vi "AlliGator Phasor Plot Actions.vi"(0 "AlliGator Q Elements in":T4[](array[typedef]), 1 "VI in":refnum<vi>, 2 "Script in":bool, 5 "data value reference in":refnum<data-value>, 7 "AlliGator Q Event in":T5=enum."GUI:Idle", 9 "Data":variant, 11 "error in (no error)":errorcluster, 12 "AlliGator Ctrl Refnums":T6) -> (3 "Script out":bool, 4 "AlliGator Q Elements out":T4[](array[typedef]), 6 "Data Value Reference out":refnum<data-value>, 10 "[Notebook Message]":T1[](array[typedef]) {"Message Style"."Text Alignment" items=["Left", "Right", "Center"]}, 15 "error out":errorcluster)   [LabVIEW 2021, in "AlliGator Action Engine.lvlib"]
doc: "Processes AlliGator phasor plot-related actions."
uses:
  AlliGator Action Engine.lvlib
  Variant/Variant to Data/Variant to Data.lvlib
  Variant/Variant to Data/Variant to [String].vi
  AlliGator Q Event.ctl
  AlliGator Q Element.ctl
  Alligator Elements Order in Action Stack.ctl
  AlliGator Add Single Action to Stack.vi
  GUI/GUI.lvlib
  AlliGator Phasor Plot.lvlib
  AlliGator Phasor Ratio.lvlib
  Variant/Variant to Data/Variant to Boolean.vi
  AlliGator Phasor Plot Color Map.lvlib
  Image/Image.lvlib
  AlliGator Source Image.lvlib
  AlliGator Files.lvlib
  Rich Text Box/Rich Text Box.lvlib
  AlliGator Internal Variables.lvlib
  Files/Files.lvlib
  AlliGator GUI.lvlib
  AlliGator Variables List.ctl
  AlliGator Globals, Variables & Constants.lvlib
  Palette/Palette.lvlib
  Image/Image Display Palette Type.ctl
  Palette/Image Palette Information.ctl
  AlliGator ROI Manager Actions.ctl
  AlliGator ROIs.lvlib
  AlliGator Settings.lvlib
  Utilities/Read-Write.ctl
  Utilities/Utilities.lvlib
  Sound/Sound.lvlib
  <vilib>/Utility/miscctls.llb/LVPoint32TypeDef.ctl
  Image/Image Control Refnum.ctl
  Image/Image Display Mouse Click Event Data.ctl
  Time/Time.lvlib
  Phasor/Phasor (g, s).ctl
  Phasor/Phasor.lvlib
  Variant/Variant to Data/Variant to String.vi
  AlliGator Phasor Plot Image ROI Storage [SGL] v3.vi
  Variant/Variant to Data/Variant to Image.vi
  793a9f64-fd61-4161-b52c-76edb5dbf837.vi
  AlliGator Add Action Array to Stack.vi
  Image/Image Control ROI Description.ctl
  AlliGator Settings List.ctl
  AlliGator Image Display Type.ctl
  Phasor/Phasor Reference Series.ctl
  Phasor/Calibration Phasor (m, phi).ctl
  <vilib>/vision/Image Controls.llb/IMAQ Image.ctl
  Image/Named ROI Description.ctl
  AlliGator Baseline Subtraction Method.ctl
  AlliGator Decay Preprocessing.lvlib
  AlliGator Decay Background Subtraction Info.ctl
  Graphs/XY Graph/XY Graph Plot Shift Method.ctl
  Graphs/XY Graph/XY Graph Add-Ons.lvlib
  Graphs/XY Graph/XY Graph Plot Shift Parameters.ctl
  AlliGator Decay Extrapolation Parameters.ctl
  AlliGator Decay Metadata v3.ctl
  AlliGator Phasor Graph.lvlib
  AlliGator Raw Phasor Plot Data v4.ctl
  AlliGator Data Series Type.ctl
  AlliGator Gate Image Set.ctl
  AlliGator FLI Dataset Type.ctl
  Phasor/Phasor Harmonic Data.ctl
  AlliGator Phasor Multi-Harmonic Data.ctl
  AlliGator Displayed Image.ctl
  Fits/IRF(X)PSED/Decay Fit Parameters & Derived Quantities List.ctl
  Fits/Fits.lvlib
  Fits/IRF(X)PSED/Decay Fit Parameters In List.ctl
  AlliGator Decay Fit Parameter Constraints 2.ctl
  AlliGator Decay Fit.lvlib
  Fits/Decay Convolution/Decay Model.ctl
  Fits/Residual Type.ctl
  Fits/IRF(X)PSED/Fit Weights Type.ctl
  Fits/Fit Calculation Method.ctl
  Fits/Non-linear Fitting Algorithm.ctl
  AlliGator Decay Fit Options & Parameters v2.ctl
  AlliGator Decay Fit Parameter Map.lvlib
  AlliGator Gate Arithmetic.ctl
  AlliGator Internal Variables v2.ctl
  AlliGator Registered Events Ctrl Refnums.ctl
  AlliGator Dataset Ctrl Refnums.ctl
  Phasor/Phasor Calibration Type.ctl
  AlliGator Phasor Graph Ctrl Refnums.ctl
  AlliGator Phasor Plot Ctrl Refnums.ctl
  AlliGator State Indicator.ctl
  AlliGator Other Ctrl Refnums.ctl
  AlliGator Image Histogram Control Refnums.ctl
  AlliGator Decay Fit Map Control Refnums.ctl
  AlliGator Ctrl Refnums.ctl
  Rich Text Box/Text Colors.ctl
  Rich Text Box/Text Formatting.ctl
  AlliGator Dataset Channel.ctl
  AlliGator Dual-Channel Datasets.lvlib
  Histograms/Histogram Bin Position.ctl
  Histograms/Histogram Window.lvlib
  Histograms/Histogram Bin Option.ctl
  Histograms/Linear Histogram Options.ctl
  AlliGator Decay Preprocessing Parameters.ctl
  Phasor/Phasor Standard Deviation Options.ctl
  Phasor/Phasor Calibration Map v2.ctl
  Fits/Non-linear Fitting Method v2.ctl
  Fits/IRF(X)PSED/Decay Fit Options v2.ctl
  Fits/IRF(X)PSED/MLE Baseline Offset Type.ctl
  Notebook/Notebook Message Object.ctl
  Notebook/Notebook.lvlib
  AlliGator Parameter Maps Data.ctl
  AlliGator Main Window Tabs.ctl
panel:
  # "see the AlliGator License on the block diagram (Ctrl+E or Window:Show Block Diagram)"
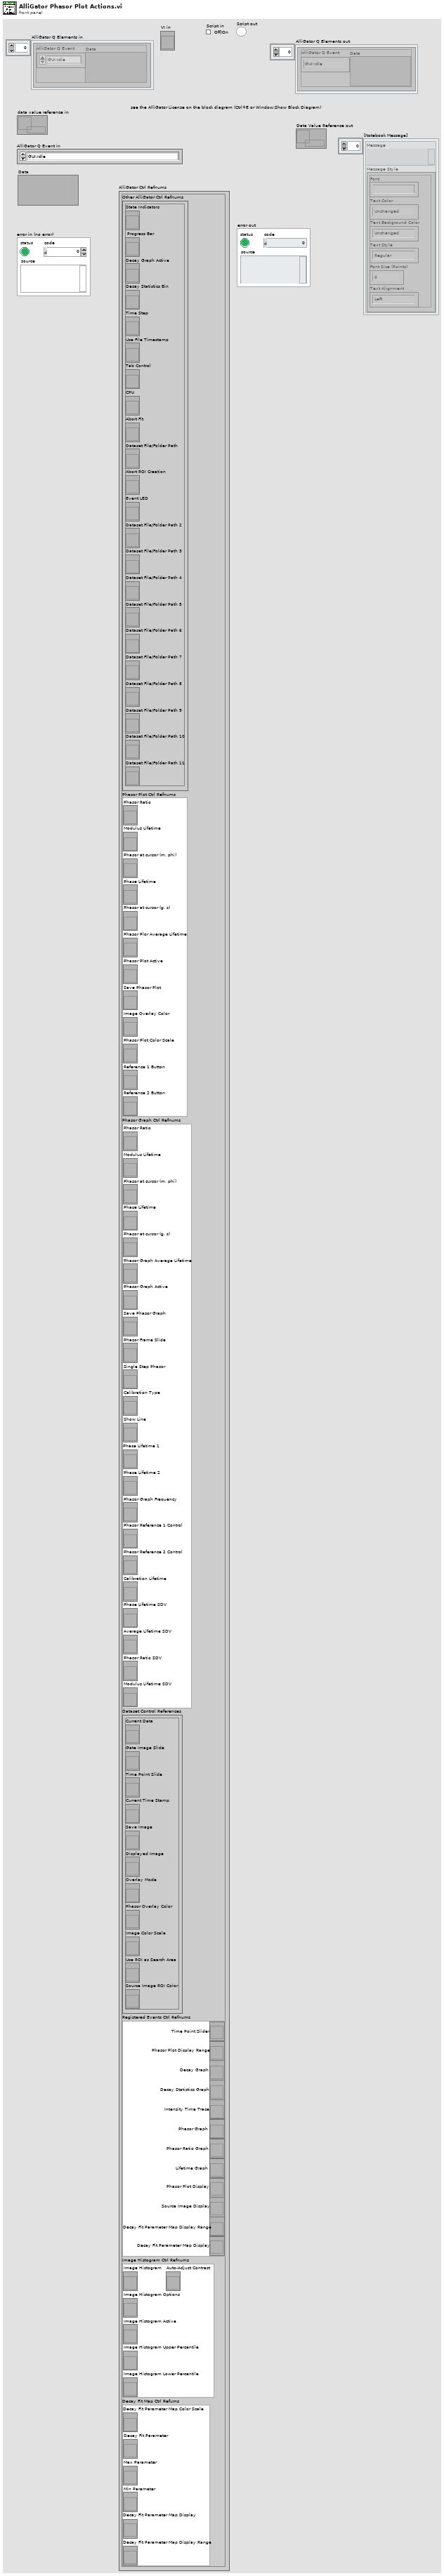
[diagram p1: front panel]
types:
  T1 = typedef "Notebook.lvlib/Notebook Message Object.ctl" = cluster{"Message":string, "Message Style":T2}
  T2 = typedef "Rich Text Box.lvlib/Text Formatting.ctl" = cluster{"Font":string, "Text Color":T3, "Text Background Color":T3, "Text Style":enum16{"Regular", "Bold", "Italic", "Underline", "Strikeout"}, "Font Size (Points)":dbl, "Text Alignment":i32}
  T3 = typedef "Rich Text Box.lvlib/Text Colors.ctl" = enum16{"Unchanged", "Black", "Blue", "Brown", "Gray", "Green", "Orange", "Pink", "Red", "White"}
  T4 = typedef "AlliGator Action Engine.lvlib/AlliGator Q Element.ctl" = cluster{"AlliGator Q Event":T5, "Data":variant}
  T5 = typedef "AlliGator Action Engine.lvlib/AlliGator Q Event.ctl" = enum16{"---- Files ----", "Files:Set Batch Export Files To Save", "Files:Set Dataset Loading & Pre-processing Options", "Files:Check #Frames in Dataset", "Files:Increment Frame Index", "Files:Open Mask Image", "Files:Open White Light Image", "Files:Open Single Dataset", "Files:New Folder of Folders Selected", "Files:Load File (all Types)_Scriptable", "Files:Move Flattened Series to Folders Series", "Files:Select Folder", "Files:Load FLI Dataset", "Files:Load Swiss SPAD 1 Dataset", "Files:Load Swiss SPAD 2 Dataset", "Files:Load .sdt FLI Dataset", "Files:Load .ptu FLI Dataset", "Files:Load .bin FLI Dataset", "Files:Load Single Gate Image Folder", "Files:Load I/m/phi Dataset (deprecated)", "Files:Load Single Image", "Files:Subtract Background File", "Files:Export FLI Dataset", "Files:Load HDF5 FLI Dataset", "Files:Set Destination File Path", "Files:Save Mask Image", "Files:Batch Conversion", "Files:New Folder Selected", "Files:Close FLI Dataset", "Files:Close FLI Dataset Series", "Files:Close White Light Image", "Files:Close Mask Image", "---- FLI Dataset ----", "FLI Dataset:Channel Arithmetic", "FLI Dataset:Export Average Lifetime Map as ASCII", "FLI Dataset:Export User-Defined Quantity Map as ASCII", "FLI Dataset:Python Function FLI Dataset Event", "FLI Dataset:ROI Analysis", "FLI Dataset:Tilted Logistic Square Gated IRF Characteristics Map", "FLI Dataset:Logistic Square Gated IRF Characteristics Map", "FLI Dataset:Square Gated IRF Characteristics Map", "FLI Dataset:Multi-ROI Single-Pixel Phasor Analysis", "FLI Dataset:Multi-ROI Single-Pixel NLSF Analysis", "FLI Dataset:All ROIs IRF Extraction", "FLI Dataset:All ROIs Decay Fit Non-Interactive (Fast + Individual IRF)", "FLI Dataset:All ROIs Phasor Analysis", "FLI Dataset:All ROIs Decay Fit", "FLI Dataset:Fluorescence Decay Statistics", "FLI Dataset:Update Decay Statistics Graph", "FLI Dataset:Get Decay from ROI", "FLI Dataset:All ROIs Average Lifetimes", "---- FLI Dataset Series ----", "FLI Dataset Series:Sum All Datasets in Series", "FLI Dataset Series:Add Dataset to Accumulated Dataset", "FLI Dataset Series:Display Accumulated Dataset", "FLI Dataset Series:Clear Dataset Series Sum", "FLI Dataset Series:Time-Series Analysis (NLSF)", "FLI Dataset Series:Time-Series Analysis (Phasor)", "---- Image ----", "Image:Update Image Profile Plots", "Image:Image Histogram Cursor Move", "Image:Image Histogram", "Image:Image Contrast", "Image:Set Image Histogram Cursor Move Flag", "Image:Clear Image Overlay", "Image:Use ROI as Search Area", "Image:Set ROI Diameter", "Image:Save Image Data as TIFF", "Image:Save Displayed Image with Overlay", "Image:Save Image Overlay Only", "Image:Save Image as Hot Pixel Mask", "Image:Change Source Image Color Palette", "Image:Copy Image to Clipboard", "Image:Source Image ROI Selection", "Image:Delete All ROIs", "Image:Delete All Unselected ROIs", "Image:Delete ROI", "Image:Merge All ROIs", "Image:Store ROI", "Image:Source Image ROI Storage", "Image:Export ROI Description to Notebook", "Image:Save ROI", "Image:Load ROI", "Image:Paste ROI Definition", "Image:Clear ROI", "Image:Identify ROIs in Mask Image", "Image:Create Complementary ROI", "Image:Create Contour ROI", "Image:Create ROI(s) from Pixels with Peak above Min_Scriptable", "Image:Create ROI(s) from Pixels with Intensity above Min_Scriptable", "Image:Compute ROI Statistics", "Image:Delete ROI(s) based on ROI Characteristics", "Image:Create ROI Grid", "Image:ROI to Individual Pixel ROIs", "Image:Python Function Source Image Event", "Image:Show Phasor Calibration Map ROI Centers", "Image:Convert ROI to Mask Image", "Image:Mouse Move", "Image:Mouse Up", "Image:Set Source Image Mouse Move Flag", "Image:Add Scale Bar Overlay", "Image:Delete Existing ROIs Option", "---- Decay ----", "Decay:Clear IRF/Reference Plot", "Decay:Clear Local IRFs", "Decay:Add Decay to Graph", "Decay:Smoothen Plot", "Decay:Smoothen Plot Tail", "Decay:Average Selected Plots", "Decay:Extract IRF", "Decay:Optimal IRF Extraction", "Decay:Threshold IRF", "Decay:Fit to Model IRF", "Decay:Fit IRF to Square Gate", "Decay:Fit IRF to Logistic Square Gate", "Decay:Fit IRF to Tilted Logistic Square Gate", "Decay:Create Bounding Cursors Set", "Decay:Export Bounding Cursors Definition to Notebook", "Decay:Denoise Plot", "Decay:Compute Cumulative Function", "Decay:Use as Reference Decay", "Decay:Show Reference Decay/IRF", "Decay:Extrapolate Decay", "Decay:Create Head & Tail Bounding Cursors", "Decay:Store Cursor-defined Head & Tail Fractions", "Decay:Rebin Plot", "Decay:1-Normalize Decay", "Decay:[0-1]-Normalize Plot", "Decay:Straighten Decay", "Decay:Shift Decay", "Decay:Fold Decay", "Decay:Fit Decay", "Decay:Global Fit of Selected Decays", "Decay:Post Global Fit Script", "Decay:Add Global Fit Parameters to Graph", "Decay:Add Decay Parameter(s) to Plot (Graph)", "Decay:Export Decay to Phasor Graph", "Decay:Plot Decay Shifts", "Decay:Compute Average Lifetime", "Decay:Plot Convolution", "Decay:Graph Tip Strip Update", "---- Decay Statistics ----", "Decay Statistics:Tip Strip Update", "---- Intensity Time Trace ----", "Intensity Time Trace:Use File Timestamp", "Intensity Time Trace:Load Intensity Corrections File", "Intensity Time Trace:Clear Intensity Corrections File", "Intensity Time Trace:Tip Strip Update", "---- Phasor Plot ----", "Phasor Plot:Build Phasor Plot", "Phasor Plot:Change Phasor Plot Color Palette", "Phasor Plot:Adjust Phasor Plot Display Range", "Phasor Plot:Highlight Image ROI in Phasor Plot", "Phasor Plot:Save Phasor Plot Image with Overlay", "Phasor Plot:Export Complex Phasor Map", "Phasor Plot:Export Phasor Ratio Map", "Phasor Plot:Export Average Lifetime Map", "Phasor Plot:Compute Phase Lifetime Histogram", "Phasor Plot:Compute Phasor Ratio Histogram", "Phasor Plot:Compute Phase Lifetime vs Intensity Scatter Plot", "Phasor Plot:Weber 2-Component Decomposition", "Phasor Plot:Update Phasor Color Map Vertices", "Phasor Plot:Clear Phasor Overlay", "Phasor Plot:Use Segment Extremities as References", "Phasor Plot:Use UC/Segment Intersections as References", "Phasor Plot:Use UC/Principal Axis Intersections as References", "Phasor Plot:Use UC/Linear Fit Intersections as References", "Phasor Plot:Update Phasor Plot Reference", "Phasor Plot:Show Local Phasor Info in Phasor Plot", "Phasor Plot:Update Phasor Plot State", "Phasor Plot:Phasor Plot ROI Storage", "Phasor Plot:Phasor Plot ROI Selection", "Phasor Plot:Python Function Phasor Plot Event", "Phasor Plot:Overlay Phasor ROI, Ratio or Map in Source Image", "Phasor Plot:Compute Decay of Selected Phasors", "Phasor Plot:Phasor at Image Pixel", "Phasor Plot:Mouse Move", "Phasor Plot:Mouse Up", "Phasor Plot:Display Range Mouse Move", "Phasor Plot:Set Mouse Move Flag", "---- Phasor Graph ----", "Phasor Graph:Calibrated Phasor Map Series", "Phasor Graph:Whole Image Phasor Scatter Plot (Todo)", "Phasor Graph:Get Phasor Value", "Phasor Graph:Create New Phasor Plot Dialog", "Phasor Graph:Update Last Phasor Value", "Phasor Graph:Update Phasor (m, phi)", "Phasor Graph:Remove Single Phasor from Plot", "Phasor Graph:Add Single Phasor to Plot", "Phasor Graph:Remove Phasor Plot", "Phasor Graph:Remove Selected Phasor Plots", "Phasor Graph:Clear Phasor Data", "Phasor Graph:Clear Phasor Graph", "Phasor Graph:Cursor Move", "Phasor Graph:Draw Cursor Connecting Line", "Phasor Graph:Clear Cursor Connecting Line", "Phasor Graph:Find UC Intersection", "Phasor Graph:Use UC/Cursor-Defined Line Intersections", "Phasor Graph:Use Selected Plots Fitted Line/UC Intersections", "Phasor Graph:Use Selected Plots Principal Axis/UC Intersections", "Phasor Graph:Show Single Phasor", "Phasor Graph:Save Single Phasor Plot", "Phasor Graph:Save All Phasor Plots", "Phasor Graph:Load Phasor Plot(s)", "Phasor Graph:Phasor Multiplication", "Phasor Graph:Compute Average Phasor", "Phasor Graph:Compute Multiple Average Phasors (Selected Plots)", "Phasor Graph:Export Single Phasor Plot Phase Lifetimes", "Phasor Graph:Phase Lifetime Trajectory", "Phasor Graph:Phase Lifetime vs Intensity Scatter Plot (deprecated)", "Phasor Graph:Parameter 2 vs Parameter 1 Scatter Plot", "Phasor Graph:Use Cursor n Location", "Phasor Graph:Set Reference n to Current Phase Lifetime Value", "Phasor Graph:Set Reference n to Lifetime Value", "Phasor Graph:Set Cursor n Location", "Phasor Graph:Save Phasor Graph Image", "Phasor Graph:Update SEPL Plot", "Phasor Graph:Export Single Phasor Plot Data", "Phasor Graph:Export Selected Phasor Plots Data", "Phasor Graph:Python Function Phasor Graph Event", "Phasor Graph:Tip Strip Update", "---- Calibration ----", "Calibration:Set Calibration Type", "Calibration:Load/Save Phasor Calibration", "Calibration:Load/Save Phasor Calibration Series", "Calibration:Load/Save Phasor Calibration Map", "Calibration:Use as Calibration", "Calibration:Compute Optimal Calibration from Phasor References", "Calibration:Clear Phasor Calibration", "Calibration:Single Phasor Calibration Information", "Calibration:Use as Calibration Series", "Calibration:Use as Calibration Map", "Calibration:Clear Calibration Series", "Calibration:Phasor Calibration Series Information", "Calibration:Clear Calibration Map", "Calibration:Phasor Calibration Map Information", "Calibration:Apply Phasor Calibration", "Calibration:Update Single Plot Calibration", "Calibration:Update Multiple Plots Calibration", "Calibration:Clear Single Plot Calibration", "Calibration:Clear All Plots Calibrations", "Calibration:Clear Plot(s) Calibration(s)?", "Calibration:Phasor Calibration Maps (# Gates Series)", "---- Phasor Ratio ----", "Phasor Ratio:Clear Reference n", "Phasor Ratio:Toggle Selected Plot(s)  Lock to Reference 1", "Phasor Ratio:Use as Reference n", "Phasor Ratio:Send Reference n to Notebook", "Phasor Ratio:Toggle Selected Plot(s)  Lock to Reference 2", "Phasor Ratio:Compute Phasor Ratio at Mouse Location", "Phasor Ratio:Compute Phasor Plot's Average Phasor Ratio", "Phasor Ratio:Compute Time-Series Phasor Ratios", "Phasor Ratio:Fit Line to Phasor Ratio Plot", "Phasor Ratio:Save References", "Phasor Ratio:Load References", "Phasor Ratio:Update Phasor Reference 1", "Phasor Ratio:Update Phasor Reference 2", "Phasor Ratio:Move Cursor n to Reference n", "Phasor Ratio:Use as Phasor Reference 1 Lifetime", "Phasor Ratio:Use as Phasor Reference 2 Lifetime", "Phasor Ratio:Export Phasor Ratio Map as ASCII", "Phasor Ratio:Tip Strip Update", "---- Lifetime & Other Parameters Graph ----", "Lifetime:Tip Strip Update", "---- Decay Fit Parameter Map ----", "Decay Fit Parameter Map:Export ROI NLSF Data as ASCII", "Decay Fit Parameter Map:Set Decay Fit  Parameter Map Selection", "Decay Fit Parameter Map:Build Decay Fit Parameter Map", "Decay Fit Parameter Map:Change Decay Fit Parameter Map Color Palette", "Decay Fit Parameter Map:Export Decay Fit Parameter Map Data as ASCII", "Decay Fit Parameter Map:Export All Decay Fit Parameter Maps Data as ASCII", "Decay Fit Parameter Map:Send Map Data to Lifetime Graph", "Decay Fit Parameter Map:Save Decay Fit Parameter Map Image", "Decay Fit Parameter Map:Save-Load IRFs & Fit Data", "Decay Fit Parameter Map:Update Local Decay Plots", "Decay Fit Parameter Map:Python Function Decay Fit Parameters Map Event", "Decay Fit Parameter Map:Overlay Decay Fit Parameter Map in Source Image", "Decay Fit Parameter Map:Plot Map Data vs Intensity", "Decay Fit Parameter Map:Mouse Up", "Decay Fit Parameter Map:Display Range Mouse Move", "---- Generic Graph ----", "Generic Graph:Generic XY Graph Event", "Generic Graph:Python Function XY Graph Event", "Generic Graph:New Plot", "Generic Graph:Save Plot", "Generic Graph:XY Plot Histogram", "Generic Graph:Set XY Graph Plot Name", "Generic Graph:Set Last Cursor Style", "Generic Graph:Tip Strip Update", "---- GUI ----", "GUI:Start Script", "GUI:Type of Displayed Image Changed", "GUI:Gate Image Slide Changed", "GUI:Show Busy Icon", "GUI:Show Busy Icon & Abort Button", "GUI:Hide Busy Icon", "GUI:Hide Busy Icon & Abort Button", "GUI:Abort", "GUI:End Script", "GUI:Start Timing", "GUI:End Timing", "GUI:Set State Indicator", "GUI:Send Parameters JSON Strings to Clipboard", "GUI:Set Gate Step", "GUI:Idle", "GUI:Initialization", "GUI:Quit", "GUI:Increment Dataset Index", "GUI:Set Dataset Index to -1", "GUI:Time Series Slider Moved", "GUI:Time Series Slider Changed", "GUI:Toggle Playback or Loop", "GUI:Playback Script", "GUI:Set Phasor Frequency", "GUI:Open Window", "GUI:Start Test Script", "GUI:End Test Script", "DEBUG"}
  T6 = typedef "AlliGator GUI.lvlib/AlliGator Ctrl Refnums.ctl" = cluster{"Other AlliGator Ctrl Refnums":T7, "Phasor Plot Ctrl Refnums":T8, "Phasor Graph Ctrl Refnums":T9, "Dataset Control References":T10, "Registered Events Ctrl Refnums":T11, "Image Histogram Ctrl Refnums":T12, "Decay Fit Map Ctrl Refums":T13}
  T7 = typedef "AlliGator GUI.lvlib/AlliGator Other Ctrl Refnums.ctl" = cluster{"State Indicators":refnum<vi>, " Progress Bar":refnum<vi>, "Decay Graph Active":refnum<vi>, "Decay Statistics Bin":refnum<vi>, "Time Step":refnum<vi>, "Use File Timestamp":refnum<vi>, "Tab Control":refnum<vi>, "CPU":refnum<vi>, "Abort Fit":refnum<vi>, "Dataset File/Folder Path":refnum<vi>, "Abort ROI Creation":refnum<vi>, "Event LED":refnum<vi>, "Dataset File/Folder Path 2":refnum<vi>, "Dataset File/Folder Path 3":refnum<vi>, "Dataset File/Folder Path 4":refnum<vi>, "Dataset File/Folder Path 5":refnum<vi>, "Dataset File/Folder Path 6":refnum<vi>, "Dataset File/Folder Path 7":refnum<vi>, "Dataset File/Folder Path 8":refnum<vi>, "Dataset File/Folder Path 9":refnum<vi>, "Dataset File/Folder Path 10":refnum<vi>, "Dataset File/Folder Path 11":refnum<vi>}
  T8 = typedef "AlliGator GUI.lvlib/AlliGator Phasor Plot Ctrl Refnums.ctl" = cluster{"Phasor Ratio":refnum<vi>, "Modulus Lifetime":refnum<vi>, "Phasor at cursor (m, phi)":refnum<vi>, "Phase Lifetime":refnum<vi>, "Phasor at cursor (g, s)":refnum<vi>, "Phasor Plor Average Lifetime":refnum<vi>, "Phasor Plot Active":refnum<vi>, "Save Phasor Plot":refnum<vi>, "Image Overlay Color":refnum<vi>, "Phasor Plot Color Scale":refnum<vi>, "Reference 1 Button":refnum<vi>, "Reference 2 Button":refnum<vi>}
  T9 = typedef "AlliGator GUI.lvlib/AlliGator Phasor Graph Ctrl Refnums.ctl" = cluster{"Phasor Ratio":refnum<vi>, "Modulus Lifetime":refnum<vi>, "Phasor at cursor (m, phi)":refnum<vi>, "Phase Lifetime":refnum<vi>, "Phasor at cursor (g, s)":refnum<vi>, "Phasor Graph Average Lifetime":refnum<vi>, "Phasor Graph Active":refnum<vi>, "Save Phasor Graph":refnum<vi>, "Phasor Frame Slide":refnum<vi>, "Single Step Phasor":refnum<vi>, "Calibration Type":refnum<vi>, "Show Line":refnum<vi>, "Phase Lifetime 1":refnum<vi>, "Phase Lifetime 2":refnum<vi>, "Phasor Graph Frequency":refnum<vi>, "Phasor Reference 1 Control":refnum<vi>, "Phasor Reference 2 Control":refnum<vi>, "Calibration Lifetime":refnum<vi>, "Phase Lifetime SDV":refnum<vi>, "Average Lifetime SDV":refnum<vi>, "Phasor Ratio SDV":refnum<vi>, "Modulus Lifetime SDV":refnum<vi>}
  T10 = typedef "AlliGator GUI.lvlib/AlliGator Dataset Ctrl Refnums.ctl" = cluster{"Current Data":refnum<vi>, "Gate Image Slide":refnum<vi>, "Time Point Slide":refnum<vi>, "Current Time Stamp":refnum<vi>, "Save Image":refnum<vi>, "Displayed Image":refnum<vi>, "Overlay Mode":refnum<vi>, "Phasor Overlay Color":refnum<vi>, "Image Color Scale":refnum<vi>, "Use ROI as Search Area":refnum<vi>, "Source Image ROI Color":refnum<vi>}
  T11 = typedef "AlliGator GUI.lvlib/AlliGator Registered Events Ctrl Refnums.ctl" = cluster{"Time Point Slider":refnum<vi>, "Phasor Plot Display Range":refnum<vi>, "Decay Graph":refnum<vi>, "Decay Statistics Graph":refnum<vi>, "Intensity Time Trace":refnum<vi>, "Phasor Graph":refnum<vi>, "Phasor Ratio Graph":refnum<vi>, "Lifetime Graph":refnum<vi>, "Phasor Plot Display":refnum<vi>, "Source Image Display":refnum<vi>, "Decay Fit Parameter Map Display Range":refnum<vi>, "Decay Fit Parameter Map Display":refnum<vi>}
  T12 = typedef "AlliGator GUI.lvlib/AlliGator Image Histogram Control Refnums.ctl" = cluster{"Image Histogram":refnum<vi>, "Image Histogram Options":refnum<vi>, "Image Histogram Active":refnum<vi>, "Image Histogram Upper Percentile":refnum<vi>, "Image Histogram Lower Percentile":refnum<vi>, "Auto-Adjust Contrast":refnum<vi>}
  T13 = typedef "AlliGator Decay Fit Parameter Map.lvlib/AlliGator Decay Fit Map Control Refnums.ctl" = cluster{"Decay Fit Parameter Map Color Scale":refnum<vi>, "Decay Fit Parameter":refnum<vi>, "Max Parameter":refnum<vi>, "Min Parameter":refnum<vi>, "Decay Fit Parameter Map Display":refnum<vi>, "Decay Fit Parameter Map Display Range":refnum<vi>}
  T14 = typedef "AlliGator Action Engine.lvlib/Alligator Elements Order in Action Stack.ctl" = enum16{"Enqueue 2 AFTER 1", "Enqueue 2 BEFORE 1"}
  T15 = typedef "Image.lvlib/AlliGator Image Display Type.ctl" = enum16{"Source Image", "Phasor Plot", "Decay Fit Parameter Map"}
  T16 = typedef "AlliGator Globals, Variables & Constants.lvlib/AlliGator Variables List.ctl" = enum16{"---- GUI ----", "GUI:Initialization Status", "GUI:State Indicators Refnum", "GUI:Original AlliGator Menu Items", "GUI:Current Action Loop State", "GUI:Script in progress", "GUI:Playback", "GUI:Loop Playback", "GUI:Search ROI Used", "GUI:Search ROI", "Decay Graph Max Legend Size", "Intensity Graph Max Legend Size", "Decay Statistics Graph Max Legend Size", "Phasor Graph Max Legend Size", "Phasor Ratio Graph Max Legend Size", "Lifetime Graph Max Legend Size", "---- Files ----", "Files:Export Dataset Frames as Individual Files", "Files:Show Batch Export Help Balloons", "Files:Frames in Dataset", "Files:ptu File Frame Start Indices", "Files:Current Frame in Dataset", "Files:Current Frame Timestamp", "Files:Dataset Loaded", "Files:Dataset Metadata", "Files:Dataset Channel", "Files:Dataset Data Description", "Files:Background Dataset Metadata", "Files:Background Dataset Channel", "Files:Background Dataset Data Description", "Files:Background File Subtraction", "Files:Background File Path", "Files:Background File Pile-up Correction", "Files:Background File Pixel Well Capacity", "Files:Background File Scaling Factor", "Files:Current Dataset Load Settings", "Files:Dataset Path", "Files:ICCD-specific Information", "Files:Macrotime Gate Separation", "------ Python Plugins ------", "Python Plugins:Information", "Python Plugins:Python Session", "Python Plugins:Valid Python Session?", "---- Source Image ----", "Source Image:ROIs", "Source Image:Current ROI", "Source Image:ROI Event Refnum", "X_Source Image Display Range", "X_Source Image Palette Information", "X_Type of Displayed Image", "X_Time Gate Slider", "Source Image:Palette List", "Source Image:Scale", "Source Image:ROI Overlay Color", "Source Image:Overlay to Erase", "Source Image:Is Displayed Image Accumulated", "---- Image Profile Window ----", "Image Profile:Overlay ROI in Source Image", "Image Profile:Window Event Refnum", "Image Profile:IntensityType", "Image Profile:Intensity Average Type", "Image Profile:Intensity-weighted SDV", "Image Profile:Box Profile Type", "Image Profile:Window Open", "Image Profile:Plotted Fit Parameter", "Source Image:White Light Image Modified", "Source Image:Mask Image Modified", "------ Phasor Graph -------", "Phasor Graph:Show Line", "---- Phasor Plot ---", "Phasor Plot:Parameters Changed", "Phasor Plot:FLI Dataset Modified since last Calculation", "Phasor Harmonics Data", "Selected Phasor Harmonics", "Phasor Harmonic Manager Event Refnum", "Phasor Plot:ROIs", "Phasor Plot::Current ROI", "Phasor Plot:ROI Event Refnum", "Phasor Plot:Image Reference Points", "Phasor Plot:Computed", "Phasor Plot:Palette Information", "Phasor Plot:Palette List", "Phasor Ratio Palette Information", "Phasor Ratio Palette List", "Phasor Plot:Image Scale", "Phasor Plot:Image Overlay to Erase", "Phasor Plot:Image Elements to Update", "Current Phasor Plot Calculation Parameters", "Current Phasor Calibration Options", "Phasor Plot:Reset Cumulated Phasor Plot", "Phasor Plot:Reference 1", "Phasor Plot:Lifetime Reference 1", "Phasor Plot:Reference 1 Frequency", "Phasor Plot:Reference 2", "Phasor Plot:Lifetime Reference 2", "Phasor Plot:Reference 2 Frequency", "---- Decay Analysis ----", "Number of Selected Decays to Fit", "LS Fit Results", "LAR Fit Results", "BS Fit Results", "Last Decay Max - Min", "Best Fit Parameters", "Best Fit Parameter Names", "Actual Size X", "Actual Size Y", "Binning X", "Binning Y", "Actual # Gates", "Dataset Number", "Gates to...", "Gates Skipped", "Gates to keep", "Gate Step", "Gate Separation", "Reversed Gates", "Pile-up Correction", "Pixel Well Capacity", "Background Subtracted", "Background Subtraction Method", "Background Definition Range", "Background File (deprecated)", "Number of Dataset Accumulated", "Array of Accumulated Dataset Paths", "Do Averaged Datasets", "Destination File Path", "Process Plot Target", "Use 1/D as Phasor Frequency", "---- Decay Fit Parameter Map -----", "Decay Fit Parameter Map Palette Information", "Decay Fit Parameter Map Palette List", "Local Decay Graph Window Event Refnum", "------- Local Decay Window ---------", "Use normalized IRF for convolution", "----- Miscellaneous ----", "Skippable Dialog Windows Status"}
  T17 = typedef "Palette.lvlib/Image Palette Information.ctl" = cluster{"Palette Name [# Colors,int?,inv?]":string, "Palette Type":T18, "Palette Colors":u32[], "Interpolate?":bool}
  T18 = typedef "Image.lvlib/Image Display Palette Type.ctl" = u32
  T19 = typedef "AlliGator Settings.lvlib/AlliGator Settings List.ctl" = enum16{"GUI:Visible Settings Tab", "GUI:Last Run Version", "Source Image:Use Image Histogram for Contrast", "Source Image:Low Count Pixels Rejection Options", "Source Image:High Count Pixels Rejection Options", "Source Image:Use Image Brightness", "Source Image:Blend Overlay with Image Background", "Source Image:Use Fixed ROI Diameter", "Source Image:ROI Diameter", "Source Image:ROI Center Color", "Source Image:Peak Threshold", "Source Image:Intensity Threshold", "Source Image:Image Binning Options", "Source Image:Image Smoothing Options", "Source Image:Image Histogram Active", "Source Image:Invert Binary Mask", "Source Image:Hot Pixel Removal", "Source Image:Overlay Analyzed ROI Center", "Source Image:Auto-Adjust Contrast", "Source Image:Histogram Lower Percentile", "Source Image:Histogram Upper Percentile", "Source Image:Save Source Image", "Source Image:Scale Bar Options", "Source Image:Image Resolution (Pixel Size)", "Source Image:Flatfield Correction", "Source Image:Show Dead Left Columns Correction", "Source Image:Dead Left Columns Correction", "Source Image:Image Pre-Processing Operations Order", "Data Information:Gate Width", "Data Information:Nanotime Gate Separation", "Data Information:Macrotime Gate Separation", "Data Information:Gate Step", "Data Information:# Gates", "Data Information:Gate Image Exposure", "Data Information:Gate Image Integration", "Data Information:Gates to Skip", "Data Information:Gates to Keep", "Data Information:Define Gates to", "Data Information:Channel Name", "Data Information:Available Channel Names", "Data Information:Channel Arithmetic", "Data Information:Background File Subtraction", "Data Information:Background File", "Data Information:Background Scaling Factor", "Data Information:Background Pile-up Correction", "Data Information:Background Pixel Well Capacity", "Data Information:Laser Period", "Data Information:SYNC Period", "Data Information:Pile-up Correction", "Data Information:Pixel Well Capacity", "Data Information:Dataset Scaling Factor", "Fluorescence Decay_Decay Pre-Processing:Reverse Gates", "Fluorescence Decay_Decay Pre-Processing:Verbose Decay Pre-Processing", "Fluorescence Decay_Decay Pre-Processing:Use Decay Pre-Processing", "Fluorescence Decay_Decay Pre-Processing:Background Subtraction", "Fluorescence Decay_Decay Pre-Processing:Background Definition Range", "Fluorescence Decay_Decay Pre-Processing:Baseline Subtraction Method", "Fluorescence Decay_Decay Pre-Processing:Decay Pre-Processing Operations Order", "Fluorescence Decay_Decay Pre-Processing:Smoothing Parameter", "Fluorescence Decay_Decay Pre-Processing:Shift Decay", "Fluorescence Decay_Decay Pre-Processing:Decay Shift Parameters", "Fluorescence Decay_Decay Pre-Processing:Fold Decay", "Fluorescence Decay_Decay Pre-Processing:# Folds", "Fluorescence Decay_Decay Pre-Processing:1-Normalize Decay", "Fluorescence Decay_Decay Pre-Processing:[0-1]-Normalize Decay", "Fluorescence Decay_Decay Pre-Processing:Smoothen Decay", "Fluorescence Decay_Decay Pre-Processing:Extrapolate Decay", "Fluorescence Decay_Decay Pre-Processing:Use Periodicity", "Fluorescence Decay_Decay Pre-Processing:Use Cursors", "Fluorescence Decay_Decay Pre-Processing:Tail Fraction", "Fluorescence Decay_Decay Pre-Processing:Head Fraction", "Fluorescence Decay_Decay Pre-Processing:Additional Points", "Fluorescence Decay_Decay Pre-Processing:Straighten Decay", "Fluorescence Decay_Decay Pre-Processing:Constant Background", "Fluorescence Decay_Decay Pre-Processing:Pixel-Normalize Decay", "Fluorescence Decay_Advanced Analysis:Extract IRF instead of Decay", "Fluorescence Decay_Advanced Analysis:IRF Extraction Options", "Fluorescence Decay_Advanced Analysis:IRF Optimization Options", "Fluorescence Decay_Advanced Analysis:Square Pulse Options", "Fluorescence Decay_Advanced Analysis:IRF Order", "Fluorescence Decay_Advanced Analysis:IRF Time Constants", "Fluorescence Decay_Advanced Analysis:Wavelet Analysis Options", "Fluorescence Decay_Advanced Analysis:Average Lifetime Options", "Fluorescence Decay_Fit Options:Fit Options", "Fluorescence Decay_Fit Options:Use Legacy Fitting Approach", "Fluorescence Decay_Fit Options:Use Data Information Laser Period", "Fluorescence Decay_Fit Parameters:Displayed Fit Parameters", "Fluorescence Decay_Fit Parameters:Fit Parameter Constraints", "Fluorescence Decay_Fit Parameters:Export Tabulated Results", "Fluorescence Decay_Fit Parameters:MLE Baseline Offset Type", "Fluorescence Decay_Fit Parameters:MLE Baseline Offset", "Fluorescence Decay_Fit Parameters:Guess Parameter Names", "Fluorescence Decay_Fit Parameters:Guess Parameter Values", "Fluorescence Decay_Fit Parameters:Guess Parameters Options", "Fluorescence Decay_Styles:Show Last Decay Only", "Fluorescence Decay_Styles:Decay Graph Color Array", "Fluorescence Decay:Decay Graph Active", "Fluorescence Decay Statistics:Min Peak Value", "Fluorescence Decay Statistics:Reject Low Decay Peak Pixels", "Fluorescence Decay Statistics:Reject High Decay Peak Pixels", "Fluorescence Decay Statistics:Max Peak Value", "Time Traces:Use File Timestamp", "Time Traces:Time Step", "Time Traces:Use Intensity Correction File", "Time Traces:Intensity Correction File", "Phasor Plot:Phasor Plot Smoothing Options", "Phasor Plot:Phasor Plot Size", "Phasor Plot:Phasor Plot Graphics Options", "Phasor Plot:Cumulative Phasor Plot", "Phasor Plot:Use Phasor Brightness", "Phasor Plot:Blend Overlay with Phasor Background", "Phasor Plot:Save Phasor Plot", "Phasor Plot:Show References", "Phasor Plot:Phasor Ratio Decay Range", "Phasor Plot:Exponential Fading", "Phasor Plot:Phasor Ratio Reference Colors", "Phasor Plot:Reference Radius", "Phasor Plot:Show Color Map Vertices", "Phasor Plot:Phasor Plot Active", "Phasor Plot:Phasor Ratio Color Map Type", "Phasor Plot:Phasor Ratio Color Map", "Phasor Plot:Phasor Ratio Display Range", "Phasor Plot:Selected Image ROI(s)", "Phasor Plot:All Image ROIs", "Phasor Plot:Selected Phasor Plot ROI(s)", "Phasor Plot:All Phasor Plot ROIs", "Phasor Plot:Phasor Ratio Color-Coded Quantity", "Phasor Plot:Store Phasor Harmonics", "Phasor Plot:Draw Reference Segment", "Phasor Plot:User-Defined Quantity", "Phasor Graph:Phasor Frequency", "Phasor Graph:Phasor Ratio Type", "Phasor Graph:Pixel-level Phasor Computation", "Phasor Graph:Save Phasor Graph", "Phasor Graph:Phasor Graph Active", "Phasor Graph:Phasor SDV Options", "Phasor Calibration:Use Backup Calibration if needed", "Phasor Graph:Define Shortest Lifetime as", "Phasor Calibration:Backup Calibration Type", "Phasor Calibration:Calibration Type", "Phasor Calibration:Calibration Lifetime", "Phasor Calibration:Calibration Map Algorithm", "Single-Exponential Phasor Locus (SEPL):Gate Parameters", "Single-Exponential Phasor Locus (SEPL):User-defined Gate", "Single-Exponential Phasor Locus (SEPL):User-defined IRF", "Single-Exponential Phasor Locus (SEPL):Phasor Parameters", "Single-Exponential Phasor Locus (SEPL):Decay & IRF Parameters", "Single-Exponential Phasor Locus (SEPL):Display Parameters", "Lifetime Analysis:Decay Analysis Parameters", "Lifetime Analysis:Lifetime Map Active", "Plugins:Python Settings", "Miscellaneous:Verbose Mode", "Miscellaneous:Beep after Script", "Miscellaneous:Saved Image File Format", "Miscellaneous:Exported Gate Image Settings", "Miscellaneous:Include Loading in Timing", "Miscellaneous:Verbose Settings Mode", "Miscellaneous:Histogram Options", "Miscellaneous:Beep on Error", "Miscellaneous:# Logical Processors Used", "Miscellaneous:ROI Description Max Characters", "Miscellaneous:Verbose Error Mode", "Miscellaneous:Transparent Mask Color"}
  T20 = typedef "Image.lvlib/Image Control ROI Description.ctl" = cluster{"Image Control Label":string, "ROI Descriptor":T21}
  T21 = typedef "ROI Descriptor" = cluster{"Global Rectangle":i32[], "Contours":cluster{"ID":enum32{"External", "Internal"}, "Type":u32, "Coordinates":i32[]}[]}
  T22 = typedef "Image.lvlib/Image Display Mouse Click Event Data.ctl" = cluster{"Image Control Refnum":T23, "Mouse Coordinates":T24}
  T23 = typedef "Image.lvlib/Image Control Refnum.ctl" = refnum<vi>
  T24 = typedef "LVPoint32TypeDef.ctl" = cluster{"Horizontal":i32, "Vertical":i32}
  T25 = typedef "AlliGator ROIs.lvlib/AlliGator ROI Manager Actions.ctl" = enum16{"Undefined", "Delete Current ROI", "Delete All Unselected ROIs", "Delete Multiple ROIs", "Delete All ROIs", "Swap ROIs", "Insert ROI", "Update Current ROI Descriptor", "Rename Current ROI", "Store New ROI", "Store Multiple ROIs", "Select Next ROI", "Select Previous ROI", "Find Selected ROI", "Show All ROIs", "Update ROI Manager Window", "Merge All ROIs", "Unmerge ROI", "Set Selected ROI by ID"}
  T26 = typedef "Utilities.lvlib/Read-Write.ctl" = enum16{"Read", "Write"}
  T27 = typedef "Phasor.lvlib/Phasor (g, s).ctl" = cluster{"g":dbl, "s":dbl}
  T28 = typedef "AlliGator GUI.lvlib/AlliGator State Indicator.ctl" = cluster{"Phasor Calibration Defined":bool, "Phasor Calibration Series Defined":bool, "Phasor Calibration Map Defined":bool, "Phasor Ratio Reference 1 Defined":bool, "Phasor Ratio Reference 2 Defined":bool, "Phasor Ratio Lifetime Reference 1 Defined ":bool, "Phasor Ratio Lifetime Reference 2 Defined":bool, "Phasor Calibration Used":bool, "Phasor Calibration Series Used":bool, "Phasor Calibration Map Used":bool, "Dataset Update Needed":bool, "Phasor Plot Update Needed":bool, "Reference/IRF Defined":bool, "Individual IRFs Defined":bool}
  T29 = typedef "Image.lvlib/Image Display User Event Data.ctl" = cluster{"Image Control Refnum":T23, "Coords":T24, "button info":cluster{"button 1":bool, "button 2":bool, "button 3":bool, "button 4":bool}, "keys pressed":enum16{"0", "1", "2", "3", "4", "5", "6", "7", "8", "9", "A", "B", "C", "D", "E", "F", "G", "H", "I", "J", "K", "L", "M", "N", "O", "P", "Q", "R", "S", "T", "U", "V", "W", "X", "Y", "Z", "F1", "F2", "F3", "F4", "F5", "F6", "F7", "F8", "F9", "F10", "F11", "F12", "F13", "F14", "F15", "ADD", "BACK", "BACKSLASH", "CAPITAL", "COMMA", "DECIMAL", "DELETE", "DIVIDE", "DOWN", "END", "EQUALS", "ESCAPE", "GRAVE (`)", "HOME", "INSERT", "LBRACKET", "LCONTROL", "LEFT", "L ALT", "LSHIFT", "LWIN", "MINUS", "MULTIPLY", "NEXT", "NUMLOCK", "NUMPAD_0", "NUMPAD_1", "NUMPAD_2", "NUMPAD_3", "NUMPAD_4", "NUMPAD_5", "NUMPAD_6", "NUMPAD_7", "NUMPAD_8", "NUMPAD_9", "PAUSE", "PERIOD", "PRIOR (PG UP)", "RBRACKET", "RCONTROL", "RETURN", "RIGHT", "R ALT", "RSHIFT", "RWIN", "SCROLL", "SEMICOLON", "SLASH", "SPACE", "SUBTRACT", "TAB", "UP", "ENTER (num pad)", "' (quote)"}[]}
  T30 = typedef "AlliGator Phasor Plot.lvlib/AlliGator Phasor Plot Mouse Up Event Data.ctl" = cluster{"Current ROI Tool":u32, "ROI Descriptor":T31, "Shift":bool, "Alt":bool}
  T31 = typedef "Image.lvlib/Image ROI Descriptor.ctl" = cluster{"Global Rectangle":i32[], "Contours":T32[]}
  T32 = typedef "Image.lvlib/Image Contour Definition.ctl" = cluster{"Contour Type":T33, "ROI Type":T34, "Points":i32[]}
  T33 = typedef "Image.lvlib/Image Contour ID.ctl" = enum32{"External", "Internal"}
  T34 = typedef "Image.lvlib/Image ROI Type.ctl" = enum16{"No Selection", "Point", "Line", "Rectangle", "Oval", "Polygon", "Freehand Region", "Annulus", "Unused2", "Unused3", "Broken Line", "Freehand Line", "Rotated Rectangle"}
  T35 = typedef "Image.lvlib/Image Color Scale Information.ctl" = cluster{"Scale.Maximum":dbl, "Scale.Minimum":dbl, "Scale.High Color":u32, "Scale.Low Color":u32}
  T36 = typedef "IMAQ Image.ctl" = refnum<image>
  T37 = cluster{"Global Rectangle":i32[], "Contours":cluster{"Contour Type":u32, "ROI Type":u32, "Points":i32[]}[]}
  T38 = typedef "Image.lvlib/Image Save File Format.ctl" = enum16{"PNG", "JPEG", "BMP"}
  T39 = typedef "Image.lvlib/Image Point.ctl" = cluster{"X":i32, "Y":i32}
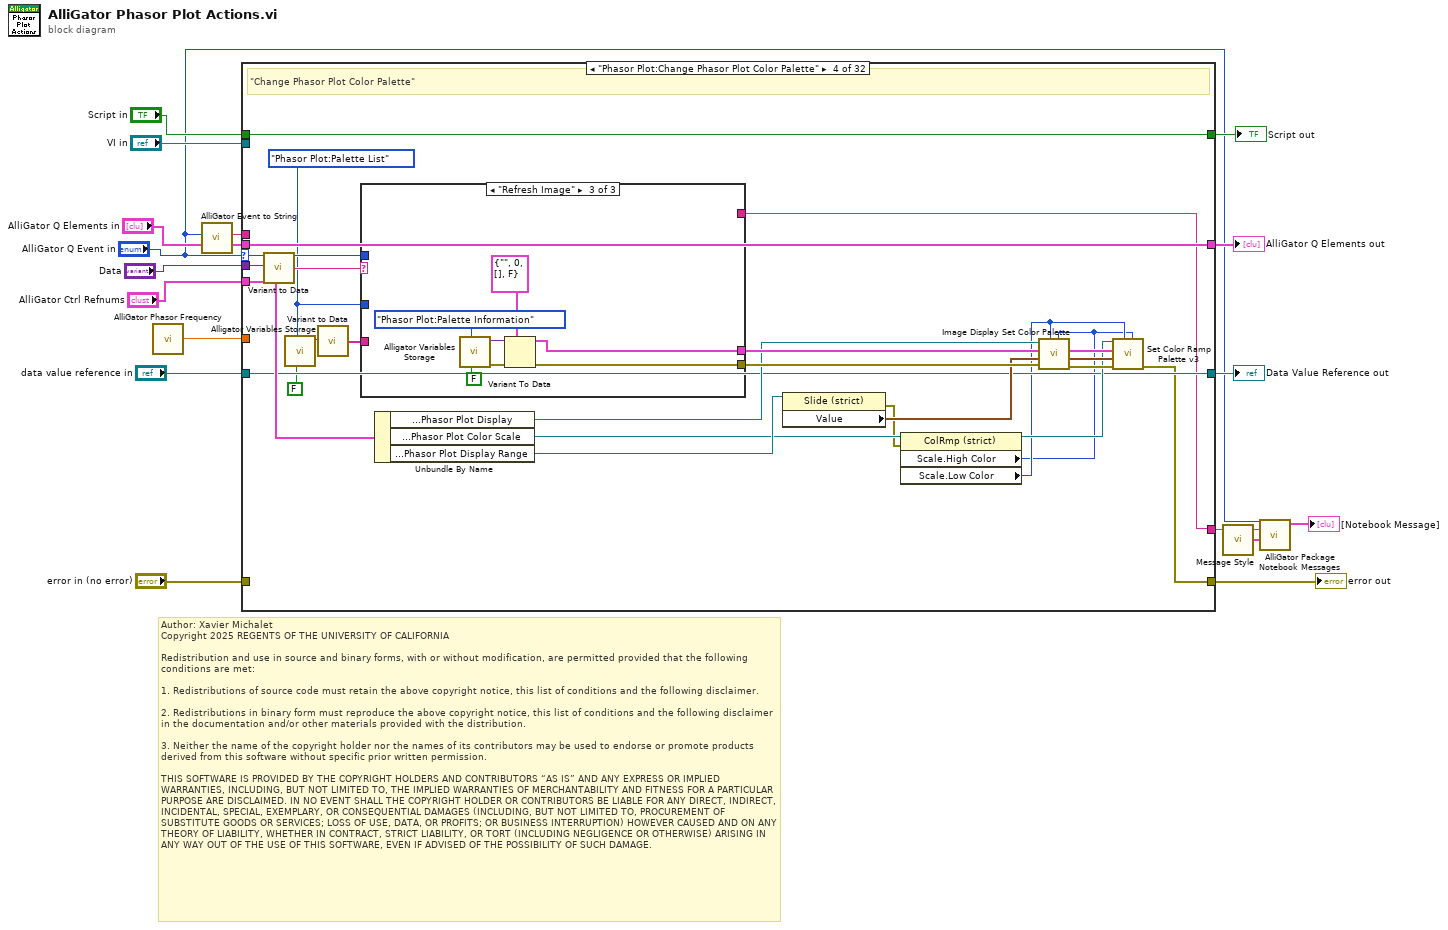
[diagram p0: block diagram]
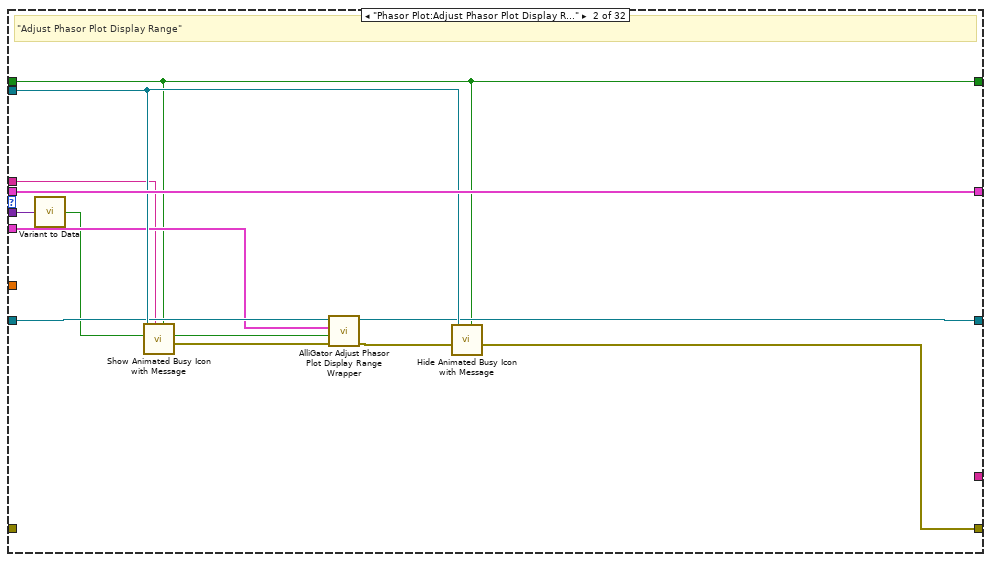
[diagram p3: hidden frame]
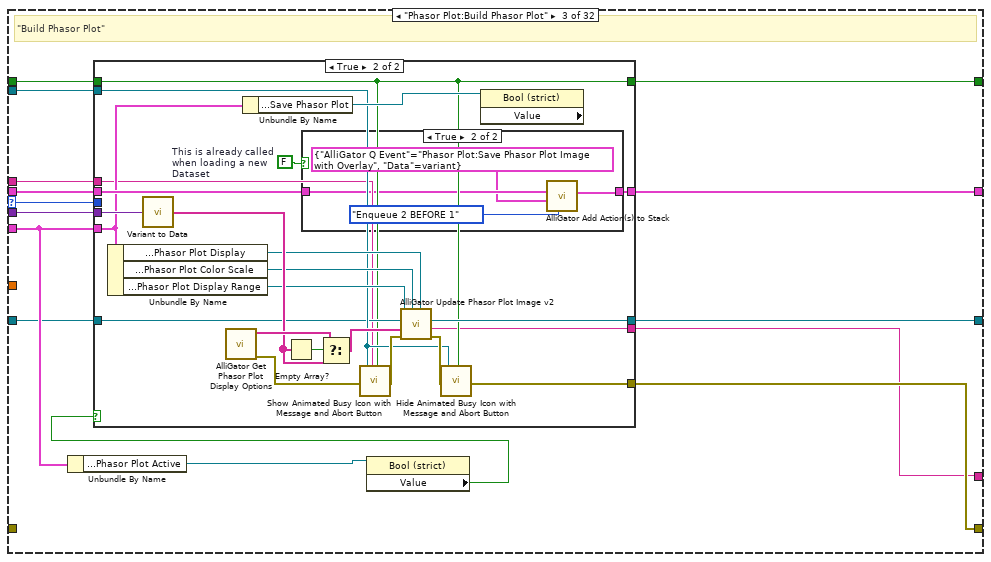
[diagram p4: hidden frame]
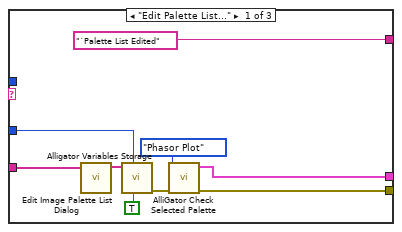
[diagram p7: hidden frame]
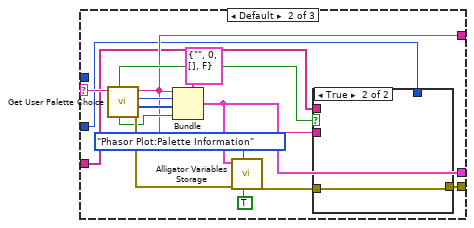
[diagram p8: hidden frame]
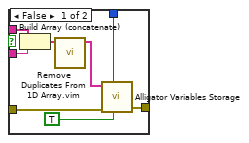
[diagram p9: hidden frame]
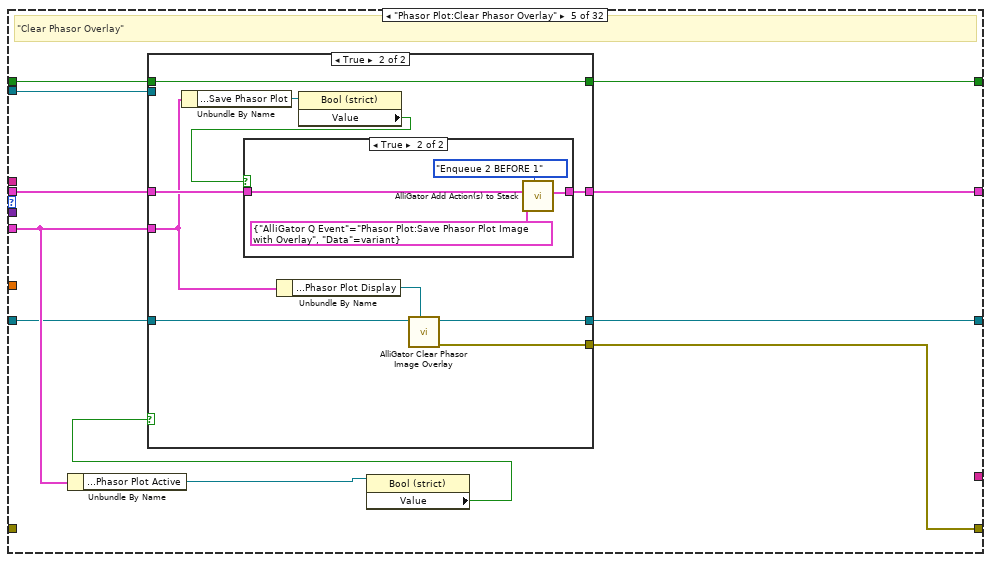
[diagram p10: hidden frame]
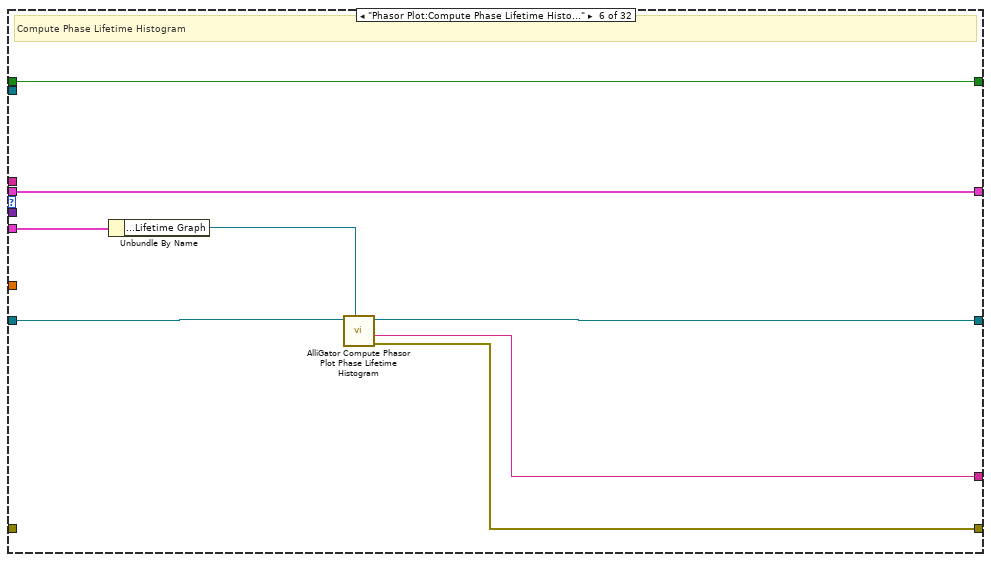
[diagram p13: hidden frame]
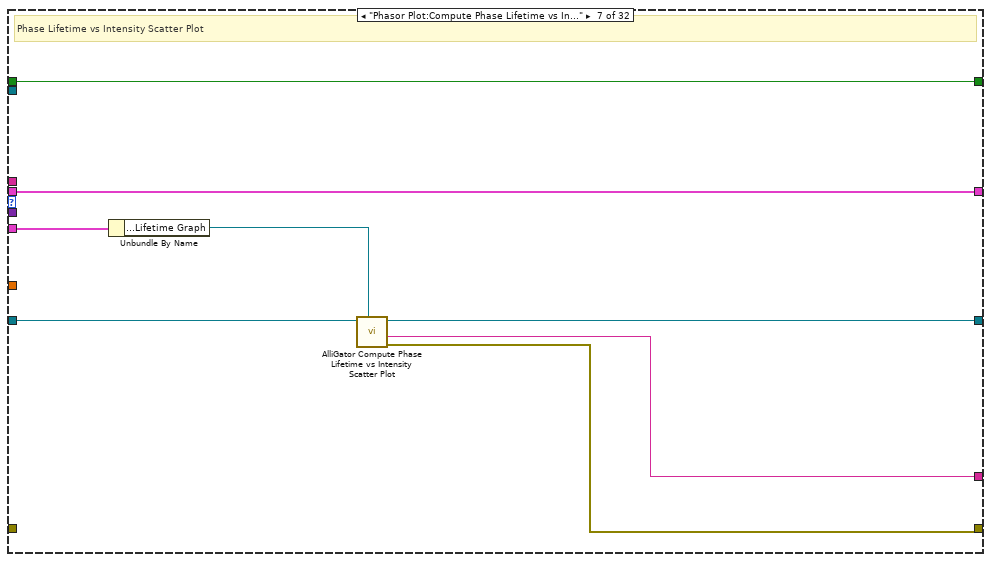
[diagram p14: hidden frame]
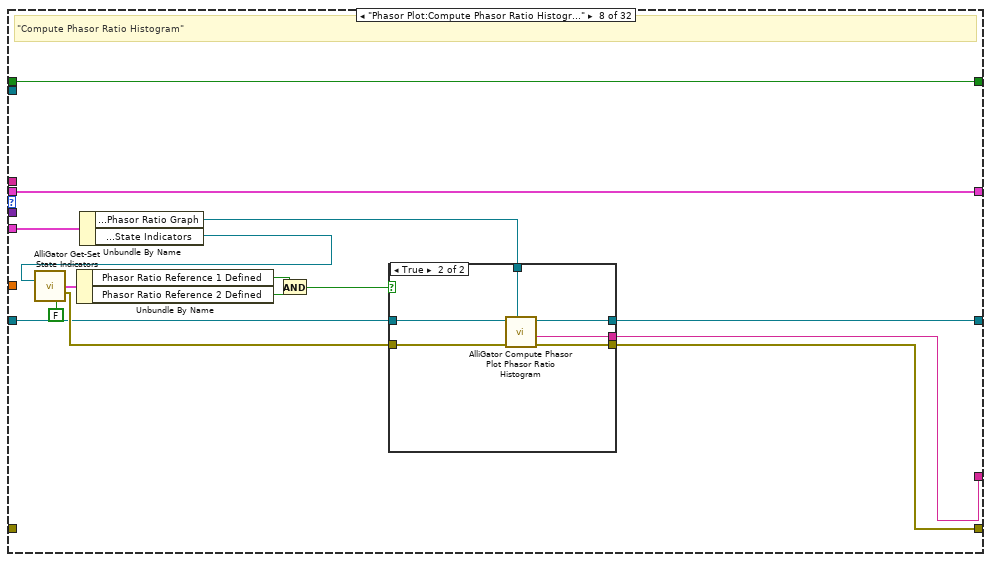
[diagram p15: hidden frame]
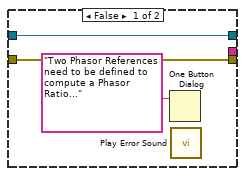
[diagram p16: hidden frame]
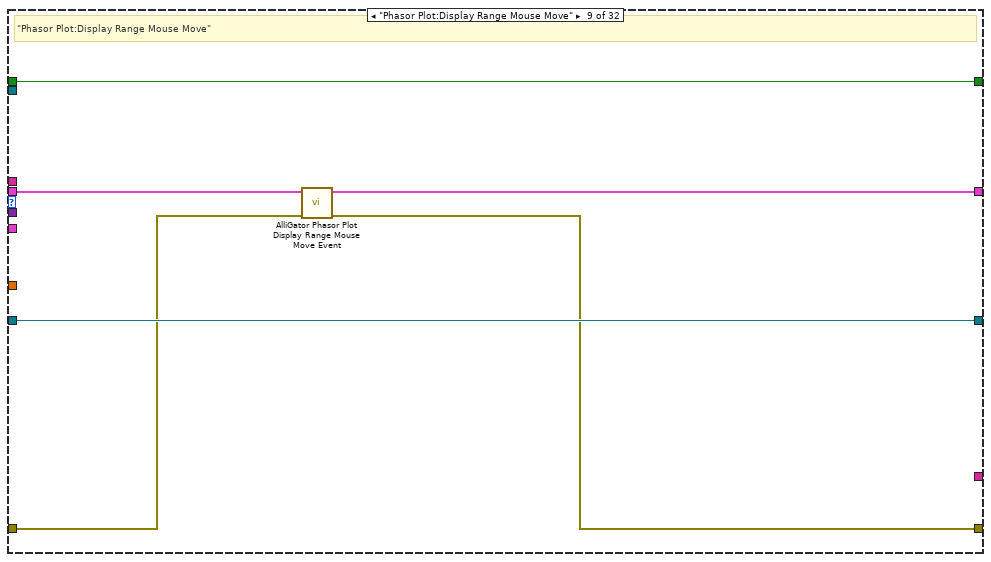
[diagram p17: hidden frame]
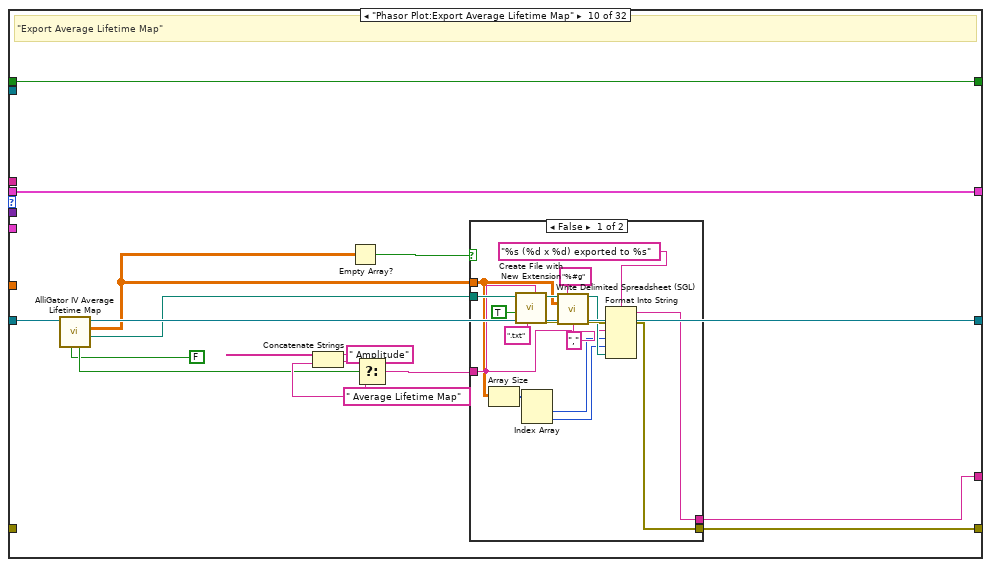
[diagram p18: hidden frame]
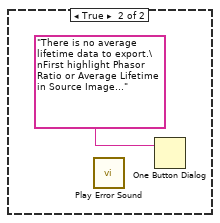
[diagram p19: hidden frame]
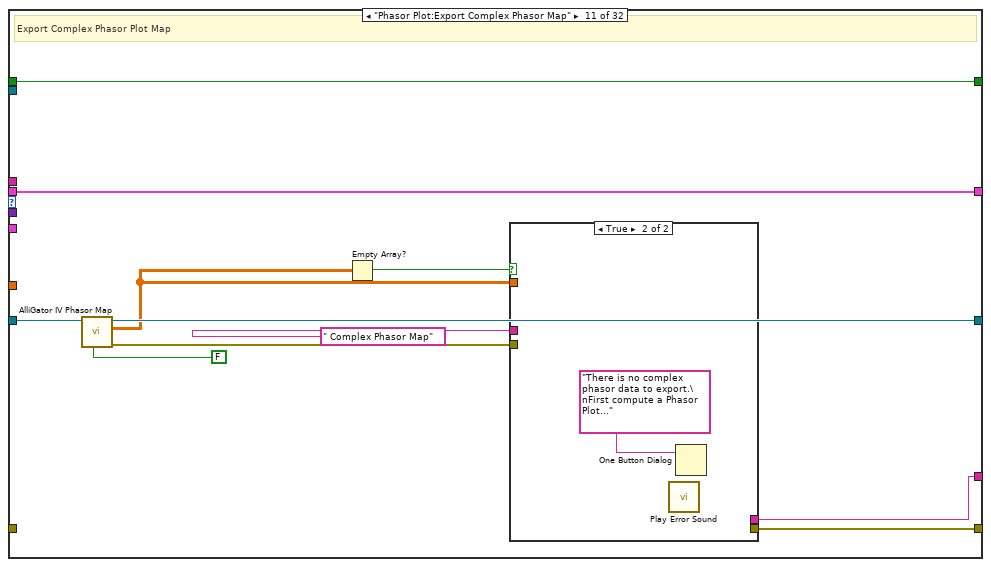
[diagram p20: hidden frame]
diagram:
  # "Author: Xavier Michalet\nCopyright 2025 REGENTS OF THE UNIVERSITY OF CALIFORNIA\n\nRedistribution and use in source and binary forms, with or without modification, are permitted provided that the following conditions are met:\n\n1. Redistributions of source code must retain the above copyright notice, this list of conditions and the following disclaimer.\n\n2. Redistributions in binary form must reproduce the above copyright notice, this list of conditions and the following disclaimer in the documentation and/or other materials provided with the distribution.\n\n3. Neither the name of the copyright holder nor the names of its contributors may be used to endorse or promote products derived from this software without specific prior written permission.\n\nTHIS SOFTWARE IS PROVIDED BY THE COPYRIGHT HOLDERS AND CONTRIBUTORS “AS IS” AND ANY EXPRESS OR IMPLIED WARRANTIES, INCLUDING, BUT NOT LIMITED TO, THE IMPLIED WARRANTIES OF MERCHANTABILITY AND FITNESS FOR A PARTICULAR PURPOSE ARE DISCLAIMED. IN NO EVENT SHALL THE COPYRIGHT HOLDER OR CONTRIBUTORS BE LIABLE FOR ANY DIRECT, INDIRECT, INCIDENTAL, SPECIAL, EXEMPLARY, OR CONSEQUENTIAL DAMAGES (INCLUDING, BUT NOT LIMITED TO, PROCUREMENT OF SUBSTITUTE GOODS OR SERVICES; LOSS OF USE, DATA, OR PROFITS; OR BUSINESS INTERRUPTION) HOWEVER CAUSED AND ON ANY THEORY OF LIABILITY, WHETHER IN CONTRACT, STRICT LIABILITY, OR TORT (INCLUDING NEGLIGENCE OR OTHERWISE) ARISING IN ANY WAY OUT OF THE USE OF THIS SOFTWARE, EVEN IF ADVISED OF THE POSSIBILITY OF SUCH DAMAGE."
  n1 = call "AlliGator Phasor Frequency.vi"() -> ("Phasor Frequency"=w12:dbl[unit])
  n2 = call "AlliGator Event to String.vi"("AlliGator Q Event"="AlliGator Q Event in") -> ("String"=w6:string)  [unwired: 8 in]
  n3 = case shown="\"Phasor Plot:Change Phasor Plot Color Palette\"" "AlliGator Q Event in" {
    selector: "AlliGator Q Event in" -> [_ _ w46 w102 _ _ _ _ _ _ _ _ _ _ _ w370 w473 _ _ _ _ _ _ _ _ _ _ _ _ _ _ _]
    tunnel: "Data" -> [_ w32 w45 w103 _ _ _ _ _ _ _ _ _ w346 w358 w369 w472 w514 w547 w566 _ w600 w605 w629 _ _ _ w688 _ w716 w732 _]
    tunnel: "AlliGator Q Elements in" -> [w21 w33 w48 w97 w154 w180 w188 w203 w216 w233 w262 w292 w323 w341 w356 w371 w474 w509 w550 w569 w574 w602 w609 w612 w643 w655 w676 w685 w703 w720 w726 w740]
    tunnel: [w21 w33 w47 w97 w153 w180 w188 w203 w215 w233 w262 w292 w322 w340 w355 w365 w468 w509 w550 w569 w574 w602 w609 w612 w642 w654 w676 w684 w700 w719 w725 w740] -> w9
    tunnel: "VI in" -> [_ w28 w44 _ w152 _ _ _ _ _ _ _ w319 _ _ w372 w475 w516 _ _ _ _ _ _ _ w653 _ _ w695 w710 _ _]
    tunnel: w12 -> [_ _ _ _ _ _ _ _ _ _ _ _ _ _ _ _ _ _ _ _ _ _ _ _ _ _ _ w679 w697 w712 w723 _]
    tunnel: "Script in" -> [w18 w23 w43 w87 w145 w173 w181 w189 w217 w219 w252 w282 w313 w347 w359 w362 w465 w507 w536 w551 w570 w580 w606 w630 w633 w652 w673 w677 w690 w705 w721 w733]
    tunnel: "error in (no error)" -> [w20 _ _ _ _ _ _ _ w213 _ _ _ _ w338 w357 _ _ w508 _ _ w573 w575 w608 w616 _ _ w675 _ _ _ _ _]
    tunnel: [w20 w30 w42 w88 w151 w175 w183 w202 w214 w232 w261 w291 w321 w339 w351 w366 w469 w510 w538 w555 w573 w590 w608 w615 w639 w651 w675 w683 w698 w717 w724 w735] -> w7
    tunnel: "AlliGator Ctrl Refnums" -> [_ w25 w40 w95 w148 w178 w186 w194 _ _ _ _ w318 w343 w350 w368 w471 w513 w540 w563 _ w592 _ w626 w638 w648 _ _ _ _ _ w738]
    tunnel: "data value reference in" -> [w19 w27 w38 w89 w146 w177 w185 w192 w218 w225 w258 w288 w315 w348 w360 w367 w470 w512 w537 w552 w572 w588 w607 w631 w637 w647 w674 w678 w694 w709 w722 w737]
    tunnel: [w19 w26 w37 w89 w147 w176 w184 w191 w218 w226 w257 w287 w316 w348 w360 w363 w466 w511 w537 w552 w572 w587 w607 w631 w636 w646 w674 w678 w693 w708 w722 w736] -> w17
    tunnel: [_ _ w34 w84 _ w174 w182 w190 _ w220 w253 w283 _ _ _ _ w463 _ _ _ _ w581 _ _ _ _ _ _ w691 w706 _ w734] -> w4
    tunnel: w6 -> [_ w22 w35 _ _ _ _ _ _ _ _ _ w314 _ _ w364 w467 w515 _ _ _ _ _ _ _ w645 _ _ w689 w704 _ _]
    tunnel: [w18 w23 w36 w87 w144 w173 w181 w189 w217 w219 w252 w282 w312 w347 w359 w361 w464 w507 w536 w551 w570 w580 w606 w630 w633 w644 w673 w677 w690 w705 w721 w733] -> w5
    frame "---- Phasor Plot ----", Default {
      # "\"---- Phaso Plot ----\""
    }
    frame "Phasor Plot:Adjust Phasor Plot Display Range" {
      # "\"Adjust Phasor Plot Display Range\""
      n4 = call-poly "Variant to Data.vi"("Variant"=w32) -> ("Value"=w24:bool)  [unwired: 8 in]
      n5 = call "Show Animated Busy Icon with Message.vi"("Already active? (F)"=w23, "Message"=w22, "Target VI Refnum"=w28) -> ("Error Out"=w29:errorcluster)  [unwired: 8 in]
      n6 = call "AlliGator Adjust Phasor Plot Display Range Wrapper.vi"("error in (no error)"=w29, "Compute Phasor Plot (T)"=w24, "AlliGator Ctrl Refnums"=w25, "Data Value Reference in"=w27) -> ("error out"=w31:errorcluster, "Data Value Reference out"=w26:refnum<data-value>)  [unwired: 6 in]
      n7 = call "Hide Animated Busy Icon with Message.vi"("Already active? (F)"=w23, "Error In"=w31, "Target VI reference"=w28) -> ("Error Out"=w30:errorcluster)  [unwired: 8 in]
    }
    frame "Phasor Plot:Build Phasor Plot" {
      # "\"Build Phasor Plot\""
      n8 = Unbundle By Name(w40) -> ("Phasor Plot Ctrl Refnums.Phasor Plot Active"=w41:refnum<vi>)
      n9 = property class="Bool (strict)"(reference=w41) -> ("Value"=w39:bool)  [unwired: 1 in, 2 out]
      n10 = case shown="True" w39 {
        tunnel: w48 -> [w51 w74]
        tunnel: [w51 w73] -> w47
        tunnel: w46 -> [_ _]
        tunnel: w45 -> [_ w70]
        tunnel: w44 -> [_ w59]
        tunnel: w43 -> [w49 w55]
        tunnel: [_ w56] -> w42
        tunnel: w40 -> [_ w61]
        tunnel: w38 -> [w50 w58]
        tunnel: [w50 w57] -> w37
        tunnel: [w49 w55] -> w36
        tunnel: w35 -> [_ w54]
        tunnel: [_ w52] -> w34
        frame False {
        }
        frame True {
          w53 = FALSE  # This is already called when loading a new Dataset
          n11 = Unbundle By Name(w61) -> ("Registered Events Ctrl Refnums.Phasor Plot Display"=w60:refnum<vi>, "Phasor Plot Ctrl Refnums.Phasor Plot Color Scale"=w63:refnum<vi>, "Registered Events Ctrl Refnums.Phasor Plot Display Range"=w64:refnum<vi>)
          n12 = call-poly "Variant to Data.vi"("Variant"=w70) -> ("String Array"=w66:string[])  [unwired: 8 in]
          n13 = call "AlliGator Get Phasor Plot Display Options.vi"() -> ("error out"=w68:errorcluster, "Phasor Plot Image Elements to Update"=w67:string[])  [unwired: 10 in]
          n14 = Unbundle By Name(w61) -> ("Phasor Plot Ctrl Refnums.Save Phasor Plot"=w62:refnum<vi>)
          n15 = Empty Array?(array=w66) -> (empty?=w69:bool)
          n16 = case shown="True" w53 {
            tunnel: w74 -> [w75 w79]
            tunnel: [w75 w78] -> w73
            frame False {
            }
            frame True {
              n17 = call-poly "AlliGator Add Action(s) to Stack.vi"("Elements Order in Action Stack (Default: 2 BEFORE 1)"=Alligator_Elements_Order_in_Action_Stack."Enqueue 2 BEFORE 1", "Alligator Atomic Action"=T4 {"AlliGator Q Event"=enum."Phasor Plot:Save Phasor Plot Image with Overlay", "Data"=variant}, "Alligator Queue Element 1"=w79) -> ("Alligator Queue Element 1 (+ 2)"=w78:T4[])  [unwired: 7 in, 1 out]
            }
          }
          n18 = Select(t=w67, s=w69, f=w66) -> (s? t:f=w65:string[])
          n19 = call "Show Animated Busy Icon with Message and Abort Button.vi"("Already active? (F)"=w55, "Message"=w54, "Target VI reference"=w59, "Error In"=w68) -> ("Error Out"=w72:errorcluster)  [unwired: 15 in]
          n20 = call "AlliGator Update Phasor Plot Image v2.vi"("Image Control Refnum"=w60, "Phasor Plot Color Scale"=w63, "Error In"=w72, "Phasor Plot Image Elements to Update"=w65, "AlliGator Internal Variables DVR"=w58, "Phasor Plot Display Range Refnum"=w64) -> ("Error Out"=w71:errorcluster, "Message"=w52:string, "AlliGator Internal Variables DVR"=w57:refnum<data-value>)  [unwired: 3 in]
          n21 = call "Hide Animated Busy Icon with Message and Abort Button.vi"("Already active? (F)"=w55, "Target VI reference"=w59, "Error In"=w71) -> ("Error Out"=w56:errorcluster)  [unwired: 16 in]
          n22 = property class="Bool (strict)" props=["Value"](reference=w62) -> ()  [unwired: 1 in, 3 out]
        }
      }
    }
    frame "Phasor Plot:Change Phasor Plot Color Palette" {
      w80 = AlliGator_Variables_List."Phasor Plot:Palette List" ("Alligator Variable")
      # "\"Change Phasor Plot Color Palette\""
      n23 = call-poly "Variant to Data.vi"("Variant"=w103) -> ("String"=w101:string)  [unwired: 8 in]
      n24 = call "Alligator Variables Storage.vi"("Get(F)/Set"=FALSE, "AlliGator Variable"=w80) -> ("Data out"=w83:variant)  [unwired: 7 in, 2 out]
      n25 = call-poly "Variant to Data.vi"("Variant"=w83) -> ("String Array"=w82:string[])  [unwired: 8 in]
      n26 = case shown="\"Refresh Image\"" w101 {
        selector: w101 -> [_ w127 _]
        tunnel: w102 -> [_ _ _]
        tunnel: [w109 w116 w139] -> w100
        tunnel: [w108 w119 w137] -> w99
        tunnel: ["`Palette List Edited" ("Append to Message") w117 _] -> w84
        tunnel: w82 -> [w105 w114 _]
        tunnel: w80 -> [w104 w113 _]
        frame "Edit Palette List..." {
          n27 = call "Edit Image Palette List Dialog.vi"("Palette List (in)"=w105) -> ("Palette List (out)"=w112:string[])  [unwired: 10 in]
          n28 = call "Alligator Variables Storage.vi"("Get(F)/Set"=TRUE, "AlliGator Variable"=w104, "Data in"=w112) -> ("Error Out"=w110:errorcluster)  [unwired: 6 in, 2 out]
          n29 = call "AlliGator Check Selected Palette.vi"("Error In"=w110, "Image"=AlliGator_Image_Display_Type."Phasor Plot") -> ("Error Out"=w109:errorcluster, "Image Display Palette Information"=w108:T17)  [unwired: 8 in]
        }
        frame Default {
          n30 = call "Get User Palette Choice.vi"("Palette"=w127) -> ("Error Out"=w122:errorcluster, "Palette Colors"=w125:u32[], "Palette Type"=w126:T18, "Palette Name (# Colors)"=w117:string, "Interpolate?"=w120:bool, "Built-in Palette?"=w118:bool)  [unwired: 3 in, 2 out]
          n31 = Bundle(cluster=T17 {"Palette Name [# Colors,int?,inv?]"="", "Palette Type"=0, "Palette Colors"=[], "Interpolate?"=FALSE} ("Image Display Palette Information"), "Palette Name [# Colors,int?,inv?]"=w117, "Palette Type"=w126, "Palette Colors"=w125, "Interpolate?"=w120) -> (w119:T17)
          n32 = call "Alligator Variables Storage.vi"("Get(F)/Set"=TRUE, "AlliGator Variable"=AlliGator_Variables_List."Phasor Plot:Palette Information" ("Alligator Variable"), "Error In"=w122, "Data in"=w119) -> ("Error Out"=w115:errorcluster)  [unwired: 5 in, 2 out]
          n33 = case shown="True" w118 {
            tunnel: w115 -> [w135 w136]
            tunnel: [w134 w136] -> w116
            tunnel: w117 -> [w133 _]
            tunnel: w114 -> [w132 _]
            tunnel: w113 -> [w130 _]
            frame False {
              n34 = Build Array (concatenate)(w132, w133) -> (w131:string[])
              n35 = call "Remove Duplicates From 1D Array.vim"("array"=w131) -> ("array with duplicates removed"=w129:string[])  [unwired: 10 in]
              n36 = call "Alligator Variables Storage.vi"("Get(F)/Set"=TRUE, "AlliGator Variable"=w130, "Error In"=w135, "Data in"=w129) -> ("Error Out"=w134:errorcluster)  [unwired: 5 in, 2 out]
            }
            frame True {
            }
          }
        }
        frame "Refresh Image" {
          n37 = call "Alligator Variables Storage.vi"("Get(F)/Set"=FALSE, "AlliGator Variable"=AlliGator_Variables_List."Phasor Plot:Palette Information" ("Alligator Variable")) -> ("Error Out"=w140:errorcluster, "Data out"=w141:variant)  [unwired: 7 in, 1 out]
          n38 = Variant To Data(error in=w140, type=T17 {"Palette Name [# Colors,int?,inv?]"="", "Palette Type"=0, "Palette Colors"=[], "Interpolate?"=FALSE} ("Image Display Palette Information"), Variant=w141) -> (data=w137:T17, error out=w139:errorcluster)
        }
      }
      n39 = Unbundle By Name(w95) -> ("Registered Events Ctrl Refnums.Phasor Plot Display"=w96:refnum<vi>, "Phasor Plot Ctrl Refnums.Phasor Plot Color Scale"=w92:refnum<vi>, "Registered Events Ctrl Refnums.Phasor Plot Display Range"=w94:refnum<vi>)
      n40 = property class="Slide (strict)"(reference=w94) -> (error out=w91:errorcluster, "Value"=w93:cluster{u32, u32})  [unwired: 1 in, 1 out]
      n41 = property class="ColRmp (strict)"(reference=w92, error in=w91) -> (reference out=w90:refnum<vi>, "Scale.High Color"=w85:u32, "Scale.Low Color"=w86:u32)  [unwired: 1 out]
      n42 = call "Image Display Set Color Palette.vi"("Image High Color"=w85, "Image Low Color"=w86, "Error In"=w100, "Image Display Range"=w93, "Image Display Palette Information"=w99, "Display Image Control Refnum"=w96) -> ("Error Out"=w98:errorcluster)  [unwired: 5 in]
      n43 = call "Set Color Ramp Palette v3.vi"("Image High Color"=w85, "Image Low Color"=w86, "error in (no error)"=w98, "Image Display Range"=w93, "Image Display Palette Information"=w99, "ColorRamp in"=w90) -> ("Error Out"=w88:errorcluster)  [unwired: 3 in, 2 out]
    }
    frame "Phasor Plot:Clear Phasor Overlay" {
      # "\"Clear Phasor Overlay\""
      n44 = Unbundle By Name(w148) -> ("Phasor Plot Ctrl Refnums.Phasor Plot Active"=w150:refnum<vi>)
      n45 = property class="Bool (strict)"(reference=w150) -> ("Value"=w149:bool)  [unwired: 1 in, 2 out]
      n46 = case shown="True" w149 {
        tunnel: w154 -> [w157 w167]
        tunnel: [w157 w166] -> w153
        tunnel: w152 -> [_ _]
        tunnel: w145 -> [w155 w158]
        tunnel: [_ w165] -> w151
        tunnel: w148 -> [_ w162]
        tunnel: w146 -> [w156 w160]
        tunnel: [w156 w159] -> w147
        tunnel: [w155 w158] -> w144
        frame False {
        }
        frame True {
          n47 = Unbundle By Name(w162) -> ("Phasor Plot Ctrl Refnums.Save Phasor Plot"=w164:refnum<vi>)
          n48 = Unbundle By Name(w162) -> ("Registered Events Ctrl Refnums.Phasor Plot Display"=w161:refnum<vi>)
          n49 = property class="Bool (strict)"(reference=w164) -> ("Value"=w163:bool)  [unwired: 1 in, 2 out]
          n50 = case shown="True" w163 {
            tunnel: w167 -> [w168 w172]
            tunnel: [w168 w171] -> w166
            frame False {
            }
            frame True {
              n51 = call-poly "AlliGator Add Action(s) to Stack.vi"("Elements Order in Action Stack (Default: 2 BEFORE 1)"=Alligator_Elements_Order_in_Action_Stack."Enqueue 2 BEFORE 1", "Alligator Atomic Action"=T4 {"AlliGator Q Event"=enum."Phasor Plot:Save Phasor Plot Image with Overlay", "Data"=variant}, "Alligator Queue Element 1"=w172) -> ("Alligator Queue Element 1 (+ 2)"=w171:T4[])  [unwired: 7 in, 1 out]
            }
          }
          n52 = call "AlliGator Clear Phasor Image Overlay.vi"("Image Control Refnum"=w161, "AlliGator IV DVR in"=w160) -> ("Error Out"=w165:errorcluster, "AlliGator IV DVR out"=w159:refnum<data-value>)  [unwired: 8 in]
        }
      }
    }
    frame "Phasor Plot:Compute Phase Lifetime Histogram" {
      # "Compute Phase Lifetime Histogram"
      n53 = Unbundle By Name(w178) -> ("Registered Events Ctrl Refnums.Lifetime Graph"=w179:refnum<vi>)
      n54 = call "AlliGator Compute Phasor Plot Phase Lifetime Histogram.vi"("Lifetime Graph refnum"=w179, "AlliGator IV DVR"=w177) -> ("error out"=w175:errorcluster, "Message"=w174:string, "AlliGator IV DVR"=w176:refnum<data-value>)  [unwired: 7 in]
    }
    frame "Phasor Plot:Compute Phase Lifetime vs Intensity Scatter Plot" {
      # "Phase Lifetime vs Intensity Scatter Plot"
      n55 = Unbundle By Name(w186) -> ("Registered Events Ctrl Refnums.Lifetime Graph"=w187:refnum<vi>)
      n56 = call "AlliGator Compute Phase Lifetime vs Intensity Scatter Plot.vi"("Lifetime Graph refnum"=w187, "AlliGator IV DVR"=w185) -> ("error out"=w183:errorcluster, "Message"=w182:string, "AlliGator IV DVR"=w184:refnum<data-value>)  [unwired: 7 in]
    }
    frame "Phasor Plot:Compute Phasor Ratio Histogram" {
      # "\"Compute Phasor Ratio Histogram\""
      n57 = Unbundle By Name(w194) -> ("Registered Events Ctrl Refnums.Phasor Ratio Graph"=w195:refnum<vi>, "Other AlliGator Ctrl Refnums.State Indicators"=w193:refnum<vi>)
      n58 = call "AlliGator Get-Set State Indicators.vi"("State Indicators Refnum"=w193, "Set (T)/Get"=FALSE) -> ("State Indicator Values"=w200:T28, "Error Out"=w196:errorcluster)  [unwired: 11 in, 1 out]
      n59 = Unbundle By Name(w200) -> ("Phasor Ratio Reference 1 Defined"=w199:bool, "Phasor Ratio Reference 2 Defined"=w198:bool)
      n60 = And(x=w199, y=w198) -> (x .and. y?=w197:bool)
      n61 = case shown="True" w197 {
        tunnel: [w206 w208] -> w202
        tunnel: w196 -> [w206 w209]
        tunnel: w195 -> [_ w212]
        tunnel: w192 -> [w204 w211]
        tunnel: [w204 w210] -> w191
        tunnel: [_ w207] -> w190
        frame False {
          n62 = One Button Dialog(message="Two Phasor References need to be defined to compute a Phasor Ratio...") -> ()  [unwired: 1 in, 1 out]
          n63 = call "Play Error Sound.vi"() -> ()  [unwired: 27 in, 1 out]
        }
        frame True {
          n64 = call "AlliGator Compute Phasor Plot Phasor Ratio Histogram.vi"("Phasor Ratio Graph refnum"=w212, "error in (no error)"=w209, "AlliGator IV DVR"=w211) -> ("error out"=w208:errorcluster, "Message"=w207:string, "AlliGator IV DVR"=w210:refnum<data-value>)  [unwired: 6 in]
        }
      }
    }
    frame "Phasor Plot:Display Range Mouse Move" {
      # "\"Phasor Plot:Display Range Mouse Move\""
      n65 = call "AlliGator Phasor Plot Display Range Mouse Move Event.vi"("Error In"=w213, "AlliGator Actions in"=w216) -> ("Error Out"=w214:errorcluster, "AlliGator Actions out"=w215:T4[])  [unwired: 8 in]
    }
    frame "Phasor Plot:Export Average Lifetime Map" {
      w227 = " Average Lifetime Map" ("input 1")
      # "\"Export Average Lifetime Map\""
      n66 = call "AlliGator IV Average Lifetime Map.vi"("Get (F)/ Set (T)"=FALSE, "AlliGator IV DVR in"=w225) -> ("Single Data Point Path"=w223:path, "[[Average Lifetime]]"=w224:sgl[][], "AlliGator IV DVR out"=w226:refnum<data-value>, "Amplitude Weighted Average Lifeitme"=w222:bool)  [unwired: 5 in, 1 out]
      n67 = Concatenate Strings(" Amplitude" ("input 1"), w227) -> (w228:string)
      n68 = Empty Array?(array=w224) -> (empty?=w231:bool)
      n69 = Select(t=w228, s=w222, f=w227) -> (s? t:f=w230:string)
      n70 = case shown="False" w231 {
        tunnel: [w247 _] -> w232
        tunnel: w223 -> [w245 _]
        tunnel: w224 -> [w237 _]
        tunnel: w230 -> [w240 _]
        tunnel: [w234 _] -> w220
        frame False {
          n71 = Array Size(array=w237) -> (size(s)=w238:i32[])
          n72 = call "Create File with New Extension.vi"("Suffix"=w240, "New File Extension"=".txt" ("New File Extension (with .)"), "Dialog?"=TRUE, "File Path in"=w245) -> ("Error Out"=w243:errorcluster, "New File Path out"=w244:path)  [unwired: 6 in]
          n73 = Index Array(array=w238) -> (element #1=w236:i32, element #2=w235:i32)  [unwired: 2 in]
          n74 = call "Write Delimited Spreadsheet (SGL).vi"("file path (dialog if empty)"=w244, "format (%.3f)"="%#g", "2D data"=w237, "error in (no error)"=w243, "delimiter (\\t)"="," ("delimiter (\\t)")) -> ("new file path (Not A Path if cancelled)"=w246:path, "error out"=w248:errorcluster)  [unwired: 9 in]
          n75 = Format Into String(format string="%s (%d x %d) exported to %s", error in=w248, w240, w236, w235, w246) -> (resulting string=w234:string, error out=w247:errorcluster)  [unwired: 1 in]
        }
        frame True {
          n76 = call "Play Error Sound.vi"() -> ()  [unwired: 27 in, 1 out]
          n77 = One Button Dialog(message="There is no average lifetime data to export.\nFirst highlight Phasor Ratio or Average Lifetime in Source Image...") -> ()  [unwired: 1 in, 1 out]
        }
      }
    }
    frame "Phasor Plot:Export Complex Phasor Map" {
      # "Export Complex Phasor Plot Map"
      n78 = call "AlliGator IV Phasor Map.vi"("Get (F)/ Set (T)"=FALSE, "AlliGator IV DVR in"=w258) -> ("error out"=w255:errorcluster, "[[CSG Phasor]]"=w256:csg[][], "AlliGator IV DVR out"=w257:refnum<data-value>)  [unwired: 7 in]
      n79 = Empty Array?(array=w256) -> (empty?=w259:bool)
      n80 = case shown="True" w259 {
        tunnel: [w263 _] -> w261
        tunnel: w256 -> [w271 _]
        tunnel: " Complex Phasor Map" ("input 1") -> [w272 _]
        tunnel: w255 -> [w266 _]
        tunnel: [w264 _] -> w253
        frame False {
          n81 = Array Size(array=w271) -> (size(s)=w268:i32[])
          n82 = call "Create File with New Extension.vi"("Suffix"=w272, "New File Extension"=".txt" ("New File Extension (with .)"), "Error In"=w266, "Dialog?"=TRUE, "File Path in"=path "") -> ("Error Out"=w275:errorcluster, "New File Path out"=w276:path)  [unwired: 5 in]
          n83 = Index Array(array=w268) -> (element #1=w270:i32, element #2=w269:i32)  [unwired: 2 in]
          n84 = call "Files Write Delimited Spreadsheet (CSL).vi"("file path (dialog if empty)"=w276, "format (%.3f)"="%#g", "2D data"=w271, "error in (no error)"=w275, "delimiter (\\t)"="," ("delimiter (\\t)")) -> ("new file path (Not A Path if cancelled)"=w277:path, "error out"=w278:errorcluster)  [unwired: 9 in]
          n85 = Format Into String(format string="%s (%d x %d) exported to %s", error in=w278, w272, w270, w269, w277) -> (resulting string=w264:string, error out=w263:errorcluster)  [unwired: 1 in]
        }
        frame True {
          n86 = call "Play Error Sound.vi"() -> ()  [unwired: 27 in, 1 out]
          n87 = One Button Dialog(message="There is no complex phasor data to export.\nFirst compute a Phasor Plot...") -> ()  [unwired: 1 in, 1 out]
        }
      }
    }
    frame "Phasor Plot:Export Phasor Ratio Map" {
      # "\"Export Phasor Ratio Map\""
      n88 = call "AlliGator IV Phasor Ratio Map.vi"("Get (F)/ Set (T)"=FALSE, "AlliGator IV DVR in"=w288) -> ("error out"=w285:errorcluster, "[[Phasor Ratio]]"=w286:sgl[][], "AlliGator IV DVR out"=w287:refnum<data-value>)  [unwired: 7 in]
      n89 = Empty Array?(array=w286) -> (empty?=w289:bool)
      n90 = case shown="True" w289 {
        tunnel: [w307 _] -> w291
        tunnel: w286 -> [w298 _]
        tunnel: " Phasor Ratio Map" ("input 1") -> [w301 _]
        tunnel: w285 -> [w295 _]
        tunnel: [w293 _] -> w283
        frame False {
          n91 = Array Size(array=w298) -> (size(s)=w299:i32[])
          n92 = call "Create File with New Extension.vi"("Suffix"=w301, "New File Extension"=".txt" ("New File Extension (with .)"), "Error In"=w295, "Dialog?"=TRUE, "File Path in"=path "") -> ("Error Out"=w304:errorcluster, "New File Path out"=w305:path)  [unwired: 5 in]
          n93 = Index Array(array=w299) -> (element #1=w297:i32, element #2=w296:i32)  [unwired: 2 in]
          n94 = call "Write Delimited Spreadsheet (SGL).vi"("file path (dialog if empty)"=w305, "format (%.3f)"="%#g", "2D data"=w298, "error in (no error)"=w304, "delimiter (\\t)"="," ("delimiter (\\t)")) -> ("new file path (Not A Path if cancelled)"=w306:path, "error out"=w308:errorcluster)  [unwired: 9 in]
          n95 = Format Into String(format string="%s (%d x %d) exported to %s", error in=w308, w301, w297, w296, w306) -> (resulting string=w293:string, error out=w307:errorcluster)  [unwired: 1 in]
        }
        frame True {
          n96 = call "Play Error Sound.vi"() -> ()  [unwired: 27 in, 1 out]
          n97 = One Button Dialog(message="There is no phasor ratio data to export.\nFirst highlight Phasor Ratio or Average Lifetime in Source Image...") -> ()  [unwired: 1 in, 1 out]
        }
      }
    }
    frame "Phasor Plot:Highlight Image ROI in Phasor Plot" {
      # "\"Highlight Image ROI in Phasor Plot\""
      n98 = Unbundle By Name(w318) -> ("Phasor Plot Ctrl Refnums.Phasor Plot Active"=w320:refnum<vi>)
      n99 = property class="Bool (strict)"(reference=w320) -> ("Value"=w317:bool)  [unwired: 1 in, 2 out]
      n100 = case shown="True" w317 {
        tunnel: w323 -> [w326 w336]
        tunnel: [w326 w336] -> w322
        tunnel: [_ w333] -> w321
        tunnel: w313 -> [w324 w327]
        tunnel: w318 -> [_ w331]
        tunnel: w319 -> [_ w332]
        tunnel: w315 -> [w325 w330]
        tunnel: [w325 w329] -> w316
        tunnel: w314 -> [_ w328]
        tunnel: [w324 w327] -> w312
        frame False {
        }
        frame True {
          n101 = call "Show Animated Busy Icon with Message.vi"("Already active? (F)"=w327, "Message"=w328, "Target VI Refnum"=w332) -> ("Error Out"=w335:errorcluster)  [unwired: 8 in]
          n102 = call "AlliGator Highlight Image ROI in Phasor Plot Wrapper.vi"("AlliGator Ctrl Refnums"=w331, "error in (no error)"=w335, "AlliGator IV DVR in"=w330) -> ("error out"=w334:errorcluster, "AlliGator IV DVR out"=w329:refnum<data-value>)  [unwired: 7 in]
          n103 = call "Hide Animated Busy Icon with Message.vi"("Already active? (F)"=w327, "Error In"=w334, "Target VI reference"=w332) -> ("Error Out"=w333:errorcluster)  [unwired: 8 in]
        }
      }
    }
    frame "Phasor Plot:Mouse Move" {
      # "\"Phasor Plot:Cursor Move\""
      n104 = Unbundle By Name(w343) -> ("Registered Events Ctrl Refnums.Source Image Display"=w337:refnum<vi>, "Phasor Plot Ctrl Refnums"=w342:T8)
      n105 = Variant To Data(error in=w338, Variant=w346) -> (data=w345:T29, error out=w344:errorcluster)  [unwired: 1 in]
      n106 = call "AlliGator Phasor Plot Mouse Move Event.vi"("Source Image Display Refnum"=w337, "Error In"=w344, "Current Phasor Plot Information Indicators"=w342, "Image User Event Data"=w345, "Alligator Queue Elements in"=w341) -> ("Error Out"=w339:errorcluster, "AlliGator Queue Elements out"=w340:T4[])  [unwired: 5 in]
    }
    frame "Phasor Plot:Mouse Up" {
      # "\"Phasor Plot:Mouse Up\""
      n107 = Unbundle By Name(w350) -> ("Phasor Plot Ctrl Refnums"=w349:T8)
      n108 = Variant To Data(error in=w357, Variant=w358) -> (data=w354:T30, error out=w353:errorcluster)  [unwired: 1 in]
      n109 = Unbundle By Name(w350) -> ("Registered Events Ctrl Refnums.Phasor Plot Display"=w352:refnum<vi>)
      n110 = call "AlliGator Phasor Plot Mouse Up Event.vi"("Current Phasor Plot Information Indicators"=w349, "error in (no error)"=w353, "Phasor Plot Mouse Up Event Data"=w354, "Phasor Plot Image Control Refnum"=w352, "AlliGator Actions in"=w356) -> ("error out"=w351:errorcluster, "AlliGator Actions out"=w355:T4[])  [unwired: 5 in]
    }
    frame "Phasor Plot:Overlay Phasor ROI, Ratio or Map in Source Image" {
      # "\"Overlay Phasor ROI, Ratio or Map in Source Image\""
      n111 = Unbundle By Name(w368) -> ("Phasor Plot Ctrl Refnums.Phasor Plot Active"=w374:refnum<vi>)
      n112 = property class="Bool (strict)"(reference=w374) -> ("Value"=w373:bool)  [unwired: 1 in, 2 out]
      n113 = case shown="True" w373 {
        tunnel: w371 -> [w377 w396]
        tunnel: [w377 w396] -> w365
        tunnel: w370 -> [_ _]
        tunnel: w372 -> [_ w387]
        tunnel: w362 -> [w375 w378]
        tunnel: [_ w395] -> w366
        tunnel: w364 -> [_ w392]
        tunnel: w368 -> [_ w391]
        tunnel: w369 -> [_ w389]
        tunnel: w367 -> [w376 w382]
        tunnel: [w376 w380] -> w363
        tunnel: [w375 w378] -> w361
        frame False {
        }
        frame True {
          n114 = Unbundle By Name(w391) -> ("Dataset Control References.Overlay Mode"=w386:refnum<vi>, "Dataset Control References.Image Color Scale"=w390:refnum<vi>, "Registered Events Ctrl Refnums.Source Image Display"=w394:refnum<vi>, "Registered Events Ctrl Refnums.Phasor Plot Display"=w393:refnum<vi>, "Phasor Plot Ctrl Refnums.Image Overlay Color"=w384:refnum<vi>)
          n115 = property class="Ring (strict)"(reference=w386) -> ("Value"=w385:u16)  [unwired: 1 in, 2 out]
          n116 = property class="ColBox"(reference=w384) -> ("Value"=w383:u32)  [unwired: 1 in, 2 out]
          n117 = call-poly "Variant to Data.vi"("Variant"=w389) -> ("Value"=w388:bool)  [unwired: 8 in]
          n118 = call "Show Animated Busy Icon with Message.vi"("Already active? (F)"=w378, "Message"=w392, "Target VI Refnum"=w387) -> ("Error Out"=w381:errorcluster)  [unwired: 8 in]
          n119 = case shown="0, Default" w385 {
            tunnel: w393 -> [_ w424 _]
            tunnel: w394 -> [w406 w435 w443]
            tunnel: w381 -> [w405 w434 w439]
            tunnel: [w402 w414 w442] -> w379
            tunnel: w382 -> [w411 w431 w441]
            tunnel: [w410 w430 w440] -> w380
            tunnel: w390 -> [w409 w437 w444]
            tunnel: w388 -> [_ w412 _]
            tunnel: w383 -> [_ w423 _]
            frame 2 {
              # "Phasor Color Map"
              n120 = property class="ImageControl"(reference=w406, error in=w405) -> (reference out=w401:refnum<vi>, error out=w398:errorcluster, "Value"=w399:variant)
              n121 = call "Get Color Scale Information.vi"("Error In"=w405, "ColorRamp in"=w409) -> ("Error Out"=w407:errorcluster, "Image Color Scale Information"=w408:T35)  [unwired: 8 in]
              n122 = call-poly "Variant to Data.vi"("Variant"=w399) -> ("Value"=w397:T36)  [unwired: 8 in]
              n123 = Merge Errors(w407, w398) -> (w404:errorcluster)
              n124 = call "AlliGator Color Map Phasor in Original Image v3.vi"("Image Color Scale Information"=w408, "Error In"=w404, "Source Image Display"=w397, "AlliGator IV DVR in"=w411) -> ("Error Out"=w403:errorcluster, "Source Image Display"=w400:T36, "AlliGator IV DVR out"=w410:refnum<data-value>)  [unwired: 4 in, 1 out]
              n125 = property class="ImageControl"(reference=w401, error in=w403, "Value"=w400) -> (error out=w402:errorcluster)  [unwired: 1 out]
            }
            frame 0, Default {
              # "Phasor ROI"
              n126 = property class="ImageControl"(reference=w424) -> (reference out=w418:refnum<vi>, error out=w415:errorcluster, "Value"=w421:variant, "ROI"=w419:T37)  [unwired: 1 in]
              n127 = property class="ImageControl"(reference=w435, error in=w434) -> (reference out=w432:refnum<vi>, error out=w425:errorcluster, "Value"=w428:variant)
              n128 = call "Get Color Scale Information.vi"("Error In"=w434, "ColorRamp in"=w437) -> ("Error Out"=w436:errorcluster, "Image Color Scale Information"=w429:T35)  [unwired: 8 in]
              n129 = call-poly "Variant to Data.vi"("Variant"=w428) -> ("Value"=w427:T36)  [unwired: 8 in]
              n130 = call-poly "Variant to Data.vi"("Variant"=w421) -> ("Value"=w420:T36)  [unwired: 8 in]
              n131 = Merge Errors(w436, w425, w415) -> (w422:errorcluster)
              n132 = call "AlliGator Highlight Phasor ROI in Original Image v3.vi"("AlliGator IV DVR in"=w431, "Image Color Scale Information"=w429, "Temp Overlay?"=w412, "Source Image Display"=w427, "Phasor Plot Image"=w420, "Phasor Plot ROI"=w419, "Error In"=w422, "Overlay Color"=w423) -> ("AlliGator IV DVR out"=w430:refnum<data-value>, "Source Image Display out"=w426:T36, "Phasor Plot Image Out"=w416:T36, "Error Out"=w417:errorcluster)  [unwired: 3 in, 1 out]
              n133 = property class="ImageControl"(reference=w432, error in=w417, "Value"=w426) -> (error out=w433:errorcluster)  [unwired: 1 out]
              n134 = property class="ImageControl"(reference=w418, error in=w417, "Value"=w416) -> (error out=w413:errorcluster)  [unwired: 1 out]
              n135 = Merge Errors(w433, w413) -> (w414:errorcluster)
            }
            frame 1 {
              # "Phasor Ratio Map"
              n136 = call "AlliGator Get Updated Phasor Ratio References.vi"("error in (no error)"=w439) -> ("error out"=w438:errorcluster)  [unwired: 8 in, 2 out]
              n137 = case shown="No Error" w438 {
                selector: w438 -> [w445 w461]
                tunnel: w444 -> [w459 _]
                tunnel: w443 -> [w457 _]
                tunnel: [w456 w461] -> w442
                tunnel: w441 -> [w454 w462]
                tunnel: [w453 w462] -> w440
                frame No Error {
                  n138 = property class="ImageControl"(reference=w457, error in=w445) -> (reference out=w455:refnum<vi>, error out=w451:errorcluster, "Value"=w452:variant)
                  n139 = call "Get Color Scale Information.vi"("Error In"=w445, "ColorRamp in"=w459) -> ("Error Out"=w458:errorcluster, "Image Color Scale Information"=w446:T35)  [unwired: 8 in]
                  n140 = call-poly "Variant to Data.vi"("Variant"=w452) -> ("Value"=w449:T36)  [unwired: 8 in]
                  n141 = Merge Errors(w458, w451) -> (w450:errorcluster)
                  n142 = call "AlliGator Overlays Phasor Ratio or Derived Quantity on Source Image v3.vi"("Image Color Scale Information"=w446, "Error In"=w450, "Source Image Display"=w449, "AlliGator IV DVR in"=w454) -> ("Error Out"=w447:errorcluster, "Source Image Display out"=w448:T36, "AlliGator IV DVR out"=w453:refnum<data-value>)  [unwired: 4 in, 1 out]
                  n143 = property class="ImageControl"(reference=w455, error in=w447, "Value"=w448) -> (error out=w456:errorcluster)  [unwired: 1 out]
                }
                frame Error {
                  n144 = One Button Dialog(message="Two valid phasor references need to be defined for this analysis...") -> ()  [unwired: 1 in, 1 out]
                }
              }
            }
          }
          n145 = call "Hide Animated Busy Icon with Message.vi"("Already active? (F)"=w378, "Error In"=w379, "Target VI reference"=w387) -> ("Error Out"=w395:errorcluster)  [unwired: 8 in]
        }
      }
    }
    frame "Phasor Plot:Compute Decay of Selected Phasors" {
      # "\"Phasor Plot:Compute Decay of Selected Phasors\""
      n146 = Unbundle By Name(w471) -> ("Phasor Plot Ctrl Refnums.Phasor Plot Active"=w477:refnum<vi>)
      n147 = property class="Bool (strict)"(reference=w477) -> ("Value"=w476:bool)  [unwired: 1 in, 2 out]
      n148 = case shown="True" w476 {
        tunnel: w474 -> [w480 w496]
        tunnel: [w480 w495] -> w468
        tunnel: w473 -> [_ _]
        tunnel: w475 -> [_ w502]
        tunnel: w465 -> [w478 w499]
        tunnel: [_ w506] -> w469
        tunnel: w467 -> [_ w504]
        tunnel: w471 -> [_ w503]
        tunnel: w472 -> [_ _]
        tunnel: w470 -> [w479 w501]
        tunnel: [w479 w500] -> w466
        tunnel: [w478 w499] -> w464
        tunnel: [_ w486] -> w463
        frame False {
        }
        frame True {
          n149 = Unbundle By Name(w503) -> ("Registered Events Ctrl Refnums.Phasor Plot Display"=w505:refnum<vi>)
          n150 = call "Show Animated Busy Icon with Message.vi"("Already active? (F)"=w499, "Message"=w504, "Target VI Refnum"=w502) -> ("Error Out"=w497:errorcluster)  [unwired: 8 in]
          n151 = property class="ImageControl"(reference=w505, error in=w497) -> (error out=w498:errorcluster, "ROI"=w494:T37)  [unwired: 1 out]
          n152 = call "AlliGator Phasor ROI to Source Image ROI.vi"("Error In"=w498, "Phasor Plot ROI"=w494, "AlliGator IV DVR in"=w501) -> ("Error Out"=w482:errorcluster, "Message"=w486:string, "Source Image ROI"=w487:T21, "AlliGator IV DVR out"=w500:refnum<data-value>)  [unwired: 4 in, 1 out]
          n153 = Bundle By Name(cluster=T20 {"Image Control Label"="Source Image", "ROI Descriptor"={"Global Rectangle"=[], "Contours"=[]}} ("Image ROI"), "ROI Descriptor"=w487) -> (w488:T20)
          n154 = call "AlliGator Settings Storage.vi"("AlliGator Settings List"=AlliGator_Settings_List."Phasor Graph:Phasor Graph Active", "Error In"=w482) -> ("Error Out"=w481:errorcluster, "Variant Data out"=w484:variant)  [unwired: 8 in]
          n155 = call-poly "Variant to Data.vi"("Variant"=w484) -> ("Value"=w483:bool)  [unwired: 8 in]
          n156 = call "AlliGator ROI Analysis Script.vi"("Error In"=w481, "Decay Graph OR Phasor Graph Active?"=w483, "Image ROI"=w488) -> ("Error Out"=w491:errorcluster, "ROI Analysis Script"=w492:T4[])  [unwired: 7 in]
          n157 = call-poly "AlliGator Add Action(s) to Stack.vi"("Elements Order in Action Stack (Default: 2 BEFORE 1)"=Alligator_Elements_Order_in_Action_Stack."Enqueue 2 BEFORE 1", "Error In"=w491, "Alligator Queue Element 2"=w492, "Alligator Queue Element 1"=w496) -> ("Error Out"=w490:errorcluster, "Alligator Queue Element 1 (+ 2)"=w495:T4[])  [unwired: 6 in]
          n158 = call "Hide Animated Busy Icon with Message.vi"("Already active? (F)"=w499, "Error In"=w490, "Target VI reference"=w502) -> ("Error Out"=w506:errorcluster)  [unwired: 8 in]
        }
      }
    }
    frame "Phasor Plot:Phasor at Image Pixel" {
      # "Phasor at Image Pixel"
      n159 = Unbundle By Name(w513) -> ("Phasor Plot Ctrl Refnums"=w522:T8)
      n160 = disable-structure shown="Enabled" {
        disable-tunnel: w514 -> [w530 w535]
        disable-tunnel: [_ w532] -> w527
        disable-tunnel: [w528 w534] -> w526
        disable-tunnel: w508 -> [_ w531]
        frame Disabled {
          n161 = Variant To Data(type=T22 {"Image Control Refnum"=refnum, "Mouse Coordinates"={"Horizontal"=0, "Vertical"=0}} ("Mouse Click Event Data"), Variant=w530) -> (error out=w528:errorcluster)  [unwired: 1 in, 1 out]
        }
        frame Enabled {
          n162 = Variant To Data(error in=w531, type=cluster{"X":i32, "Y":i32} {"X"=0, "Y"=0} ("Last Mouse Position:All Elements"), Variant=w535) -> (data=w532:cluster{"X":i32, "Y":i32}, error out=w534:errorcluster)
        }
      }
      n163 = call "Show Animated Busy Icon with Message.vi"("Already active? (F)"=w507, "Message"=w515, "Error In"=w526, "Target VI Refnum"=w516) -> ("Error Out"=w520:errorcluster)  [unwired: 7 in]
      n164 = call "High Resolution Timing.vi"("Error In"=w520) -> ("elapsed (relative) seconds"=w517:dbl, "Error Out"=w519:errorcluster)  [unwired: 16 in, 1 out]
      n165 = call "AlliGator Get Phasor at Source Image Cursor Location.vi"("error in (no error)"=w519, "AlliGator IV DVR in"=w512, "Mouse Coordinates"=w527) -> ("Error Out"=w521:errorcluster, "Valid Location"=w523:bool, "AlliGator IV DVR out"=w511:refnum<data-value>, "Phasor"=w524:T27)  [unwired: 5 in]
      n166 = call "AlliGator Update Phasor Plot Information at Mouse Location.vi"("Error In"=w521, "Valid?"=w523, "Phasor"=w524, "Current Phasor Plot Information Indicators"=w522) -> ("Error Out"=w525:errorcluster)  [unwired: 6 in, 1 out]
      n167 = call "High Resolution Timing.vi"("relative seconds (NaN)"=w517, "Error In"=w525) -> ("Error Out"=w518:errorcluster)  [unwired: 15 in, 2 out]
      n168 = call "Hide Animated Busy Icon with Message.vi"("Already active? (F)"=w507, "Error In"=w518, "Target VI reference"=w516) -> ("Error Out"=w510:errorcluster)  [unwired: 8 in]
    }
    frame "Phasor Plot:Phasor Plot ROI Selection" {
      # "\"Phasor Plot ROI Selection\""
      n169 = Unbundle By Name(w540) -> ("Registered Events Ctrl Refnums.Phasor Plot Display"=w539:refnum<vi>)
      n170 = Bundle("Action"=AlliGator_ROI_Manager_Actions."Show All ROIs", -1) -> (w544:cluster{"Action":T25, i32})  [unwired: 1 in]
      n171 = Variant To Data(type=w544, Variant=w547) -> (data=w549:cluster{"Action":T25, i32}, error out=w548:errorcluster)  [unwired: 1 in]
      n172 = call "AlliGator Select Phasor Plot ROI.vi"("Error In"=w548, "ROI Selection Data"=w549) -> ("Error Out"=w542:errorcluster, "ROI Descriptor"=w543:T21)  [unwired: 7 in, 1 out]
      n173 = call "Image Display Get-Set ROI.vi"("Get(F)/Set"=TRUE ("Get(F)/Set(T)"), "Error In"=w542, "ROI Descriptor in"=w543, "Image Display Refnum"=w539) -> ("Error Out"=w538:errorcluster)  [unwired: 3 in, 4 out]
    }
    frame "Phasor Plot:Phasor Plot ROI Storage" {
      # "\"Phasor Plot ROI Storage\""
      n174 = Unbundle By Name(w563) -> ("Registered Events Ctrl Refnums.Phasor Plot Display"=w562:refnum<vi>)
      n175 = Variant To Data(type=AlliGator_ROI_Manager_Actions."Show All ROIs" ("Action"), Variant=w566) -> (data=w565:T25, error out=w561:errorcluster)  [unwired: 1 in]
      n176 = call "Image Display Get-Set ROI.vi"("Get(F)/Set"=FALSE ("Get(F)/Set(T)"), "Error In"=w561, "Image Display Refnum"=w562) -> ("Error Out"=w553:errorcluster, "ROI Descriptor out"=w554:T21, "Image Display Refnum (dup)"=w559:T23)  [unwired: 4 in, 2 out]
      n177 = call "ROI to Default ROI Name.vi"("Error In"=w553, "ROI"=w554) -> ("Error Out"=w568:errorcluster, "ROI Type String"=w567:string)  [unwired: 8 in]
      n178 = call-poly "AlliGator Phasor Plot Image ROI Storage [PM].vi"("Error In"=w568, "Current ROI Descriptor"=w554, "Default Name (\"ROI\")"=w567, "Action"=w565) -> ("Error Out"=w556:errorcluster, "Current ROI Descriptor"=w557:T21)  [unwired: 2 in, 4 out]
      n179 = call "Image Display Get-Set ROI.vi"("Get(F)/Set"=TRUE ("Get(F)/Set(T)"), "Error In"=w556, "ROI Descriptor in"=w557, "Image Display Refnum"=w559) -> ("Error Out"=w555:errorcluster)  [unwired: 3 in, 4 out]
    }
    frame "Phasor Plot:Python Function Phasor Plot Event" {
      # "\"Phasor Plot:Python Function Phasor Plot Event\""
      n180 = One Button Dialog(message="Not yet supported....") -> ()  [unwired: 1 in, 1 out]
      n181 = call "Play Error Sound.vi"() -> ()  [unwired: 27 in, 1 out]
    }
    frame "Phasor Plot:Save Phasor Plot Image with Overlay" {
      # "\"Save Phasor Plot Image with Overlay\""
      n182 = call-poly "Variant to Data.vi"("Variant"=w600) -> ("Value"=w599:bool)  [unwired: 8 in]
      n183 = call "AlliGator IV Dataset Path.vi"("Get (F)/ Set (T)"=FALSE, "error in (no error)"=w575, "AlliGator IV DVR in"=w588) -> ("error out"=w582:errorcluster, "[Time-Series Path]"=w585:path[], "Single Data Point Path"=w586:path, "AlliGator IV DVR out"=w587:refnum<data-value>, "Current Dataset"=w584:i32)  [unwired: 4 in]
      n184 = Unbundle By Name(w592) -> ("Registered Events Ctrl Refnums.Phasor Plot Display"=w601:refnum<vi>)
      n185 = call "AlliGator Get Image File Format.vi"("Error In"=w582) -> ("error out"=w578:errorcluster, "Transparent Mask Color"=w579:u32, "File Extension (.xxx)"=w593:string, "Image File Format"=w594:T38)  [unwired: 7 in]
      n186 = call "AlliGator Get Image Destination File Path.vi"("Image File Extension"=w593, "Image Name Prefix"="Phasor Plot " ("string"), "Error In"=w578, "Current Data Set"=w584, "Time-Series Paths"=w585, "Single Data Point Path"=w586) -> ("Error Out"=w577:errorcluster, "Image File Path"=w598:path)  [unwired: 4 in]
      n187 = call "Image File Dialog (Optional).vi"("Dialog?"=w599, "Error In"=w577, "Image File Format in"=w594, "Default file path in"=w598) -> ("Error Out"=w595:errorcluster, "Image File Format out"=w596:T38, "file path out"=w597:path)  [unwired: 5 in]
      n188 = call "Image Display Save Image.vi"("Mask Color (Transparent)"=w579, "error in (no error)"=w595, "Saved Image File Format"=w596, "File Path in"=w597, "Display Image Control Refnum"=w601) -> ("Error Out"=w590:errorcluster, "File Path out"=w589:path)  [unwired: 5 in]
      n189 = Format Into String(format string="Phasor plot Image saved with overlay to %s", w589) -> (resulting string=w581:string)  [unwired: 2 in, 1 out]
    }
    frame "Phasor Plot:Set Mouse Move Flag" {
      # "\"Phasor Plot:Set Mouse Move Flag\""
      n190 = call-poly "Variant to Data.vi"("Variant"=w605) -> ("Value"=w604:bool)  [unwired: 8 in]
      n191 = call "AlliGator Phasor Plot Mouse Move Flag.vi"("Flag (in)"=w604, "Read/Write"=Read-Write."Write") -> ()  [unwired: 7 in, 1 out]
    }
    frame "Phasor Plot:Show Local Phasor Info in Phasor Plot" {
      w624 = 0  # Reference n
      n192 = Unbundle By Name(w626) -> ("Phasor Plot Ctrl Refnums"=w621:T8)
      n193 = Bundle("Current Phasor"=T27 {"g"=nan, "s"=nan}, "Reference n"=w624) -> (w623:cluster{"Current Phasor":T27, "Reference n":i32})  [unwired: 1 in]
      n194 = Variant To Data(error in=w616, type=w623, Variant=w629) -> (data=w628:cluster{"Current Phasor":T27, "Reference n":i32}, error out=w627:errorcluster)
      n195 = Unbundle By Name(w628) -> ("Reference n"=w613:i32, "Current Phasor"=w622:T27)
      n196 = Unbundle By Name(w621) -> ("Reference 1 Button"=w620:refnum<vi>, "Reference 2 Button"=w619:refnum<vi>)
      n197 = call "AlliGator Show Local Phasor Info in Phasor Plot.vi"("error in (no error)"=w627, "Last Mouse Position"=w622, "Current Phasor Plot Information Indicators"=w621) -> ("error out"=w618:errorcluster)  [unwired: 8 in]
      n198 = case shown="2" w613 {
        tunnel: [_ TRUE ("Value")] -> w610
        frame 2 {
        }
        frame 1, Default {
        }
      }
      n199 = Not(x=w610) -> (.not. x?=w611:bool)
      n200 = property class="Bool (strict)"(reference=w619, error in=w618, "Value"=w611, "Visible"=w611) -> (error out=w617:errorcluster)  [unwired: 1 out]
      n201 = property class="Bool (strict)"(reference=w620, error in=w618, "Value"=w610, "Visible"=w610) -> (error out=w614:errorcluster)  [unwired: 1 out]
      n202 = Merge Errors(w614, w617) -> (w615:errorcluster)
    }
    frame "Phasor Plot:Update Phasor Color Map Vertices" {
      # "\"Update Phasor Color Map Vertices\""
      n203 = Unbundle By Name(w638) -> ("Registered Events Ctrl Refnums.Phasor Plot Display"=w635:refnum<vi>)
      n204 = call "AlliGator Update Phasor Color Map Vertices Wrapper.vi"("Image Control Refnum"=w635, "AlliGator IV DVR in"=w637) -> ("error out"=w634:errorcluster, "AlliGator IV DVR out"=w636:refnum<data-value>)  [unwired: 8 in]
      n205 = call-poly "AlliGator Add Action(s) to Stack.vi"("Elements Order in Action Stack (Default: 2 BEFORE 1)"=Alligator_Elements_Order_in_Action_Stack."Enqueue 2 BEFORE 1", "Error In"=w634, "Alligator Atomic Action"=T4 {"AlliGator Q Event"=enum."Phasor Plot:Overlay Phasor ROI, Ratio or Map in Source Image", "Data"=variant}, "Alligator Queue Element 1"=w643) -> ("Error Out"=w639:errorcluster, "Alligator Queue Element 1 (+ 2)"=w642:T4[])  [unwired: 6 in]
    }
    frame "Phasor Plot:Update Phasor Plot Reference" {
      # "\"Update Phasor Plot Reference\""
      n206 = Unbundle By Name(w648) -> ("Phasor Plot Ctrl Refnums.Phasor Plot Active"=w650:refnum<vi>)
      n207 = property class="Bool (strict)"(reference=w650) -> ("Value"=w649:bool)  [unwired: 1 in, 2 out]
      n208 = case shown="True" w649 {
        tunnel: w655 -> [w658 w672]
        tunnel: [w658 w672] -> w654
        tunnel: w653 -> [_ w669]
        tunnel: w652 -> [w656 w663]
        tunnel: [_ w671] -> w651
        tunnel: w648 -> [_ w668]
        tunnel: [w657 w667] -> w646
        tunnel: w647 -> [w657 w666]
        tunnel: w645 -> [_ w664]
        tunnel: [w656 w663] -> w644
        frame False {
        }
        frame True {
          n209 = Unbundle By Name(w668) -> ("Registered Events Ctrl Refnums.Phasor Plot Display"=w665:refnum<vi>)
          n210 = call "Show Animated Busy Icon with Message.vi"("Already active? (F)"=w663, "Message"=w664, "Target VI Refnum"=w669) -> ("Error Out"=w670:errorcluster)  [unwired: 8 in]
          n211 = call "AlliGator Draw Phasor Ratio Reference Overlay Wrapper.vi"("Image Control Refnum"=w665, "error in (no error)"=w670, "AlliGator IV DVR in"=w666) -> ("error out"=w662:errorcluster, "AlliGator IV DVR out"=w667:refnum<data-value>)  [unwired: 7 in]
          n212 = call "AlliGator Get-Set Phasor Plot Reference is Updated.vi"("Set/Get (F)"=TRUE, "error in (no error)"=w662, "Phasor Plot Reference Updated"=TRUE) -> ("error out"=w661:errorcluster)  [unwired: 7 in, 1 out]
          n213 = call "Hide Animated Busy Icon with Message.vi"("Already active? (F)"=w663, "Error In"=w661, "Target VI reference"=w669) -> ("Error Out"=w671:errorcluster)  [unwired: 8 in]
        }
      }
    }
    frame "Phasor Plot:Update Phasor Plot State" {
      # "UNUSED"
      # "\"Update Phasor Plot State\""
    }
    frame "Phasor Plot:Use Segment Extremities as References" {
      # "\"Use Segment Extremities as References\""
      n214 = Variant To Data(Variant=w688) -> (data=w686:T39[], error out=w687:errorcluster)  [unwired: 2 in]
      n215 = call "AlliGator Use Phasor Plot Segment Extremities as References.vi"("Error In"=w687, "Phasor Frequency"=w679, "Image Points"=w686) -> ("error out"=w680:errorcluster, "Phasor 2"=w681:T27, "Phasor 1"=w682:T27)  [unwired: 6 in]
      n216 = call "AlliGator Update Phasor Ratio References.vi"("Error In"=w680, "Phasor Reference 2"=w681, "Phasor Reference 1"=w682, "AlliGator Q Element in"=w685) -> ("error out"=w683:errorcluster, "Alligator Queue Elements out"=w684:T4[])  [unwired: 6 in]
    }
    frame "Phasor Plot:Use UC/Linear Fit Intersections as References" {
      # "\"Phasor Plot: Use UC/Linear Fit Intersections as References\""
      n217 = call "Show Animated Busy Icon with Message.vi"("Already active? (F)"=w690, "Message"=w689, "Target VI Refnum"=w695) -> ("Error Out"=w696:errorcluster)  [unwired: 8 in]
      n218 = call "AlliGator Use Phasor Plot UC-Linear Fit Intersections as References.vi"("Error In"=w696, "Phasor Frequency"=w697, "AlliGator IV DVR in"=w694) -> ("error out"=w699:errorcluster, "Phasor 2"=w701:T27, "Phasor 1"=w702:T27, "AlliGator IV DVR out"=w693:refnum<data-value>, "Message"=w691:string)  [unwired: 4 in]
      n219 = call "Hide Animated Busy Icon with Message.vi"("Already active? (F)"=w690, "Error In"=w699, "Target VI reference"=w695) -> ("Error Out"=w692:errorcluster)  [unwired: 8 in]
      n220 = call "AlliGator Update Phasor Ratio References.vi"("Error In"=w692, "Phasor Reference 2"=w701, "Phasor Reference 1"=w702, "AlliGator Q Element in"=w703) -> ("error out"=w698:errorcluster, "Alligator Queue Elements out"=w700:T4[])  [unwired: 6 in]
    }
    frame "Phasor Plot:Use UC/Principal Axis Intersections as References" {
      # "\"Use UC/Principal Axis Intersections as References\""
      n221 = call-poly "Variant to Data.vi"("Variant"=w716) -> ("Value"=w713:bool)  [unwired: 8 in]
      n222 = call "Show Animated Busy Icon with Message.vi"("Already active? (F)"=w705, "Message"=w704, "Target VI Refnum"=w710) -> ("Error Out"=w711:errorcluster)  [unwired: 8 in]
      n223 = call "AlliGator Use Phasor Plot UC-Principal Axis Intersections as References.vi"("Phasor Frequency"=w712, "Error In"=w711, "Major Axis?"=w713, "AlliGator IV DVR in"=w709) -> ("error out"=w718:errorcluster, "Phasor 2"=w714:T27, "Phasor 1"=w715:T27, "AlliGator IV DVR out"=w708:refnum<data-value>, "Message"=w706:string)  [unwired: 3 in]
      n224 = call "Hide Animated Busy Icon with Message.vi"("Already active? (F)"=w705, "Error In"=w718, "Target VI reference"=w710) -> ("Error Out"=w707:errorcluster)  [unwired: 8 in]
      n225 = call "AlliGator Update Phasor Ratio References.vi"("Error In"=w707, "Phasor Reference 2"=w714, "Phasor Reference 1"=w715, "AlliGator Q Element in"=w720) -> ("error out"=w717:errorcluster, "Alligator Queue Elements out"=w719:T4[])  [unwired: 6 in]
    }
    frame "Phasor Plot:Use UC/Segment Intersections as References" {
      # "\"Use UC/Segment Intersections as References\""
      n226 = Variant To Data(Variant=w732) -> (data=w730:T39[], error out=w731:errorcluster)  [unwired: 2 in]
      n227 = call "AlliGator Use Phasor Plot UC-Segment Intersections as References.vi"("Error In"=w731, "Phasor Frequency"=w723, "Image Points"=w730) -> ("error out"=w729:errorcluster, "Point 2"=w727:T27, "Point 1"=w728:T27)  [unwired: 6 in]
      n228 = call "AlliGator Update Phasor Ratio References.vi"("Error In"=w729, "Phasor Reference 2"=w727, "Phasor Reference 1"=w728, "AlliGator Q Element in"=w726) -> ("error out"=w724:errorcluster, "Alligator Queue Elements out"=w725:T4[])  [unwired: 6 in]
    }
    frame "Phasor Plot:Weber 2-Component Decomposition" {
      # "2-Component Decomposition"
      n229 = Unbundle By Name(w738) -> ("Registered Events Ctrl Refnums.Lifetime Graph"=w739:refnum<vi>)
      n230 = call "AlliGator Compute Phasor Plot Weber 2-Component Decomposition.vi"("Lifetime Graph refnum"=w739, "AlliGator IV DVR"=w737) -> ("error out"=w735:errorcluster, "Message"=w734:string, "AlliGator IV DVR"=w736:refnum<data-value>)  [unwired: 7 in]
    }
  }
  "Data Value Reference out" <- w17
  "error out" <- w7
  "AlliGator Q Elements out" <- w9
  "Script out" <- w5
  n231 = call "Message Style.vi"() -> ("Message Formatting"=w3:T2)
  n232 = call "AlliGator Package Notebook Messages.vi"("Message Formatting"=w3, "Message"=w4, "AlliGator Q Event in"="AlliGator Q Event in") -> ("[Notebook Message]"=→"[Notebook Message]":T1[])  [unwired: 8 in]
